vi "MAIN_load_previous_acquisition_data.vi"(3 "error in":errorcluster, 5 "Path to the saving folder":path=path "D:/MFM experiments") -> (0 "error out":errorcluster, 1 "Data cluster":T1, 2 "Menu names cluster":T2)   [LabVIEW 2015]
uses:
  GLOBAL/Global_MAIN.vi
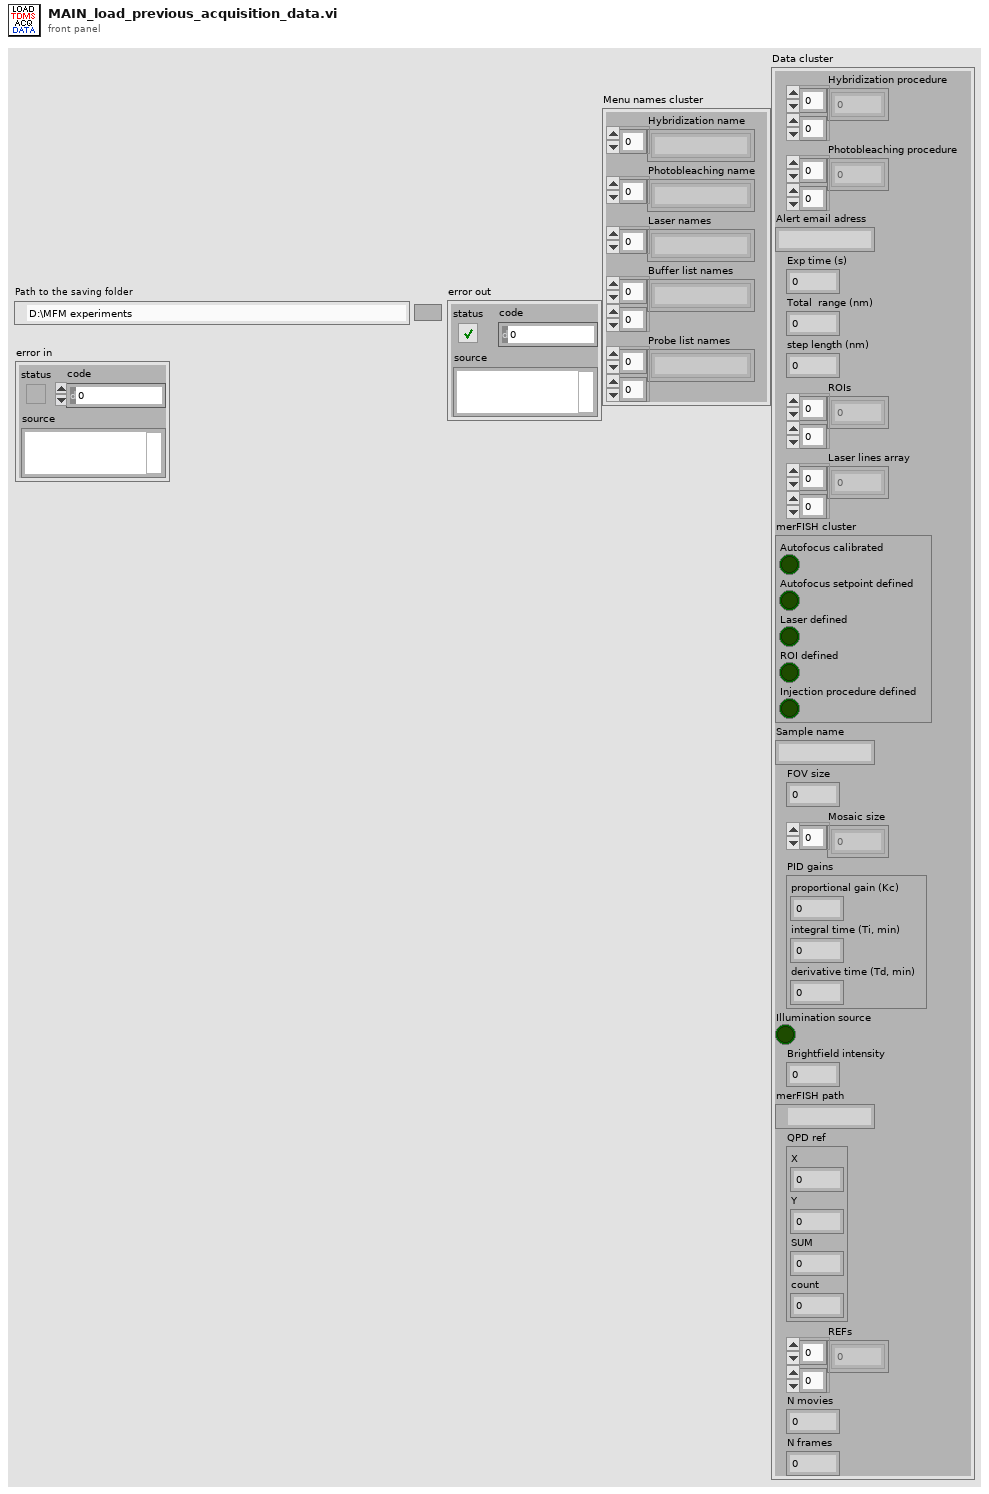
[diagram p1: front panel]
types:
  T1 = cluster{"Hybridization procedure":i32[][], "Photobleaching procedure":i32[][], "Alert email adress":string, "Exp time (s)":sgl, "Total  range (nm)":u32, "step length (nm)":u32, "ROIs":dbl[][], "Laser lines array":dbl[][], "merFISH cluster":cluster{"Autofocus calibrated":bool, "Autofocus setpoint defined":bool, "Laser defined":bool, "ROI defined":bool, "Injection procedure defined":bool}, "Sample name":string, "FOV size":dbl, "Mosaic size":u16[], "PID gains":cluster{"proportional gain (Kc)":dbl, "integral time (Ti, min)":dbl, "derivative time (Td, min)":dbl}, "Illumination source":bool, "Brightfield intensity":dbl, "merFISH path":path, "QPD ref":cluster{"X":sgl, "Y":sgl, "SUM":sgl, "count":u32}, "REFs":dbl[][], "N movies":i32, "N frames":i32}
  T2 = cluster{"Hybridization name":string[], "Photobleaching name":string[], "Laser names":string[], "Buffer list names":string[][], "Probe list names":string[][]}
  T3 = cluster{"X":sgl, "Y":sgl, "SUM":sgl, "count":u32}
  T4 = cluster{"proportional gain (Kc)":dbl, "integral time (Ti, min)":dbl, "derivative time (Td, min)":dbl}
  T5 = cluster{"Autofocus calibrated":bool, "Autofocus setpoint defined":bool, "Laser defined":bool, "ROI defined":bool, "Injection procedure defined":bool}
  T6 = enum16{"open", "open or create", "create or replace", "create", "open (read-only)"}
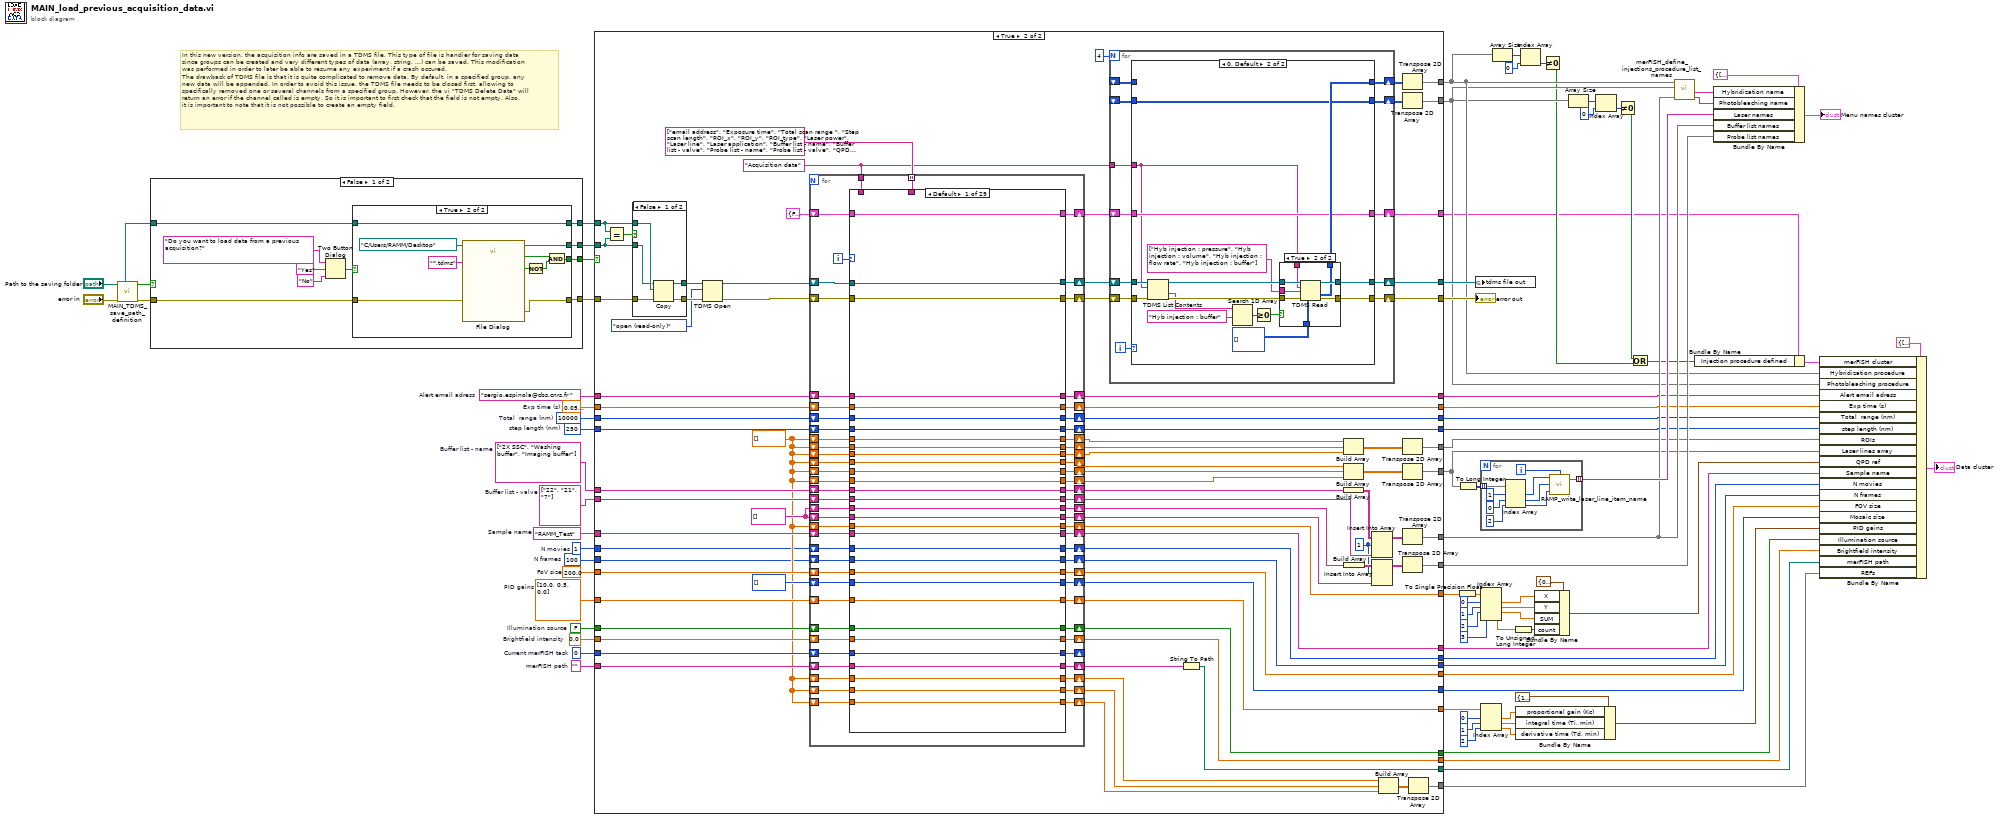
[diagram p0: block diagram]
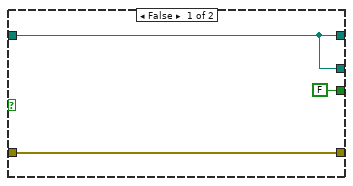
[diagram p2: hidden frame]
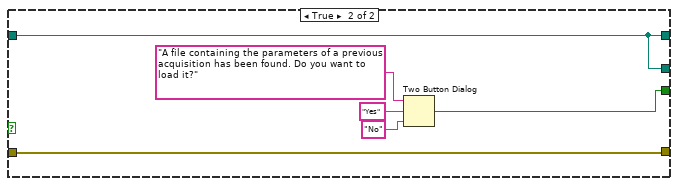
[diagram p3: hidden frame]
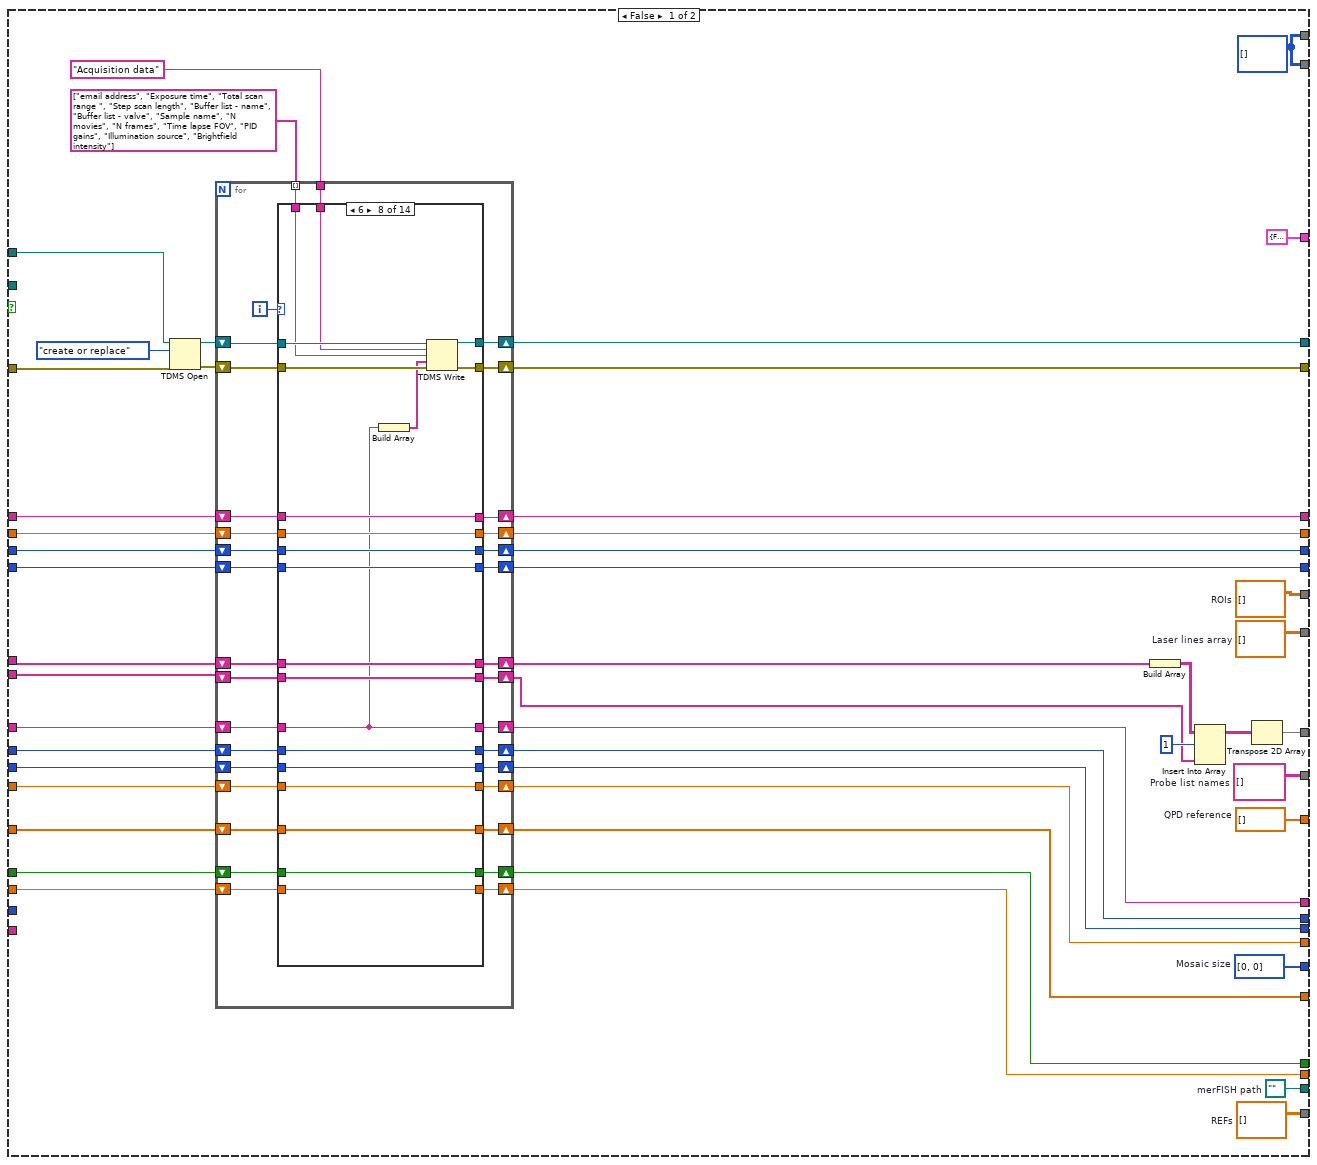
[diagram p4: hidden frame]
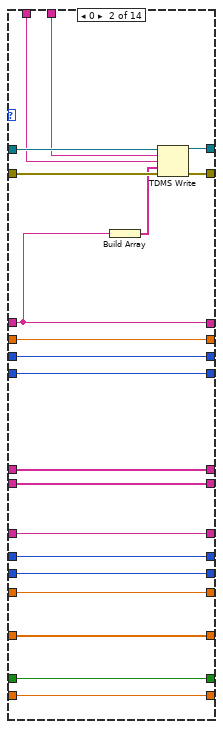
[diagram p6: hidden frame]
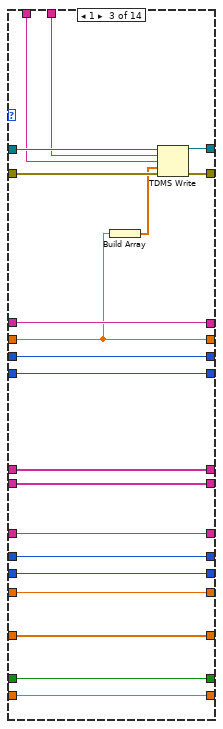
[diagram p7: hidden frame]
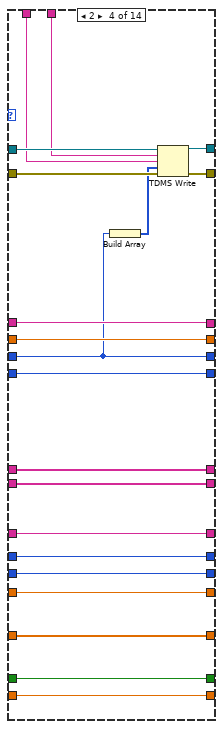
[diagram p8: hidden frame]
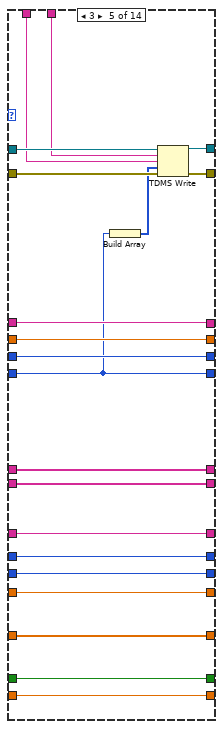
[diagram p9: hidden frame]
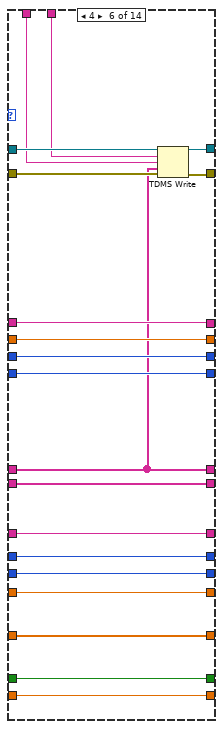
[diagram p10: hidden frame]
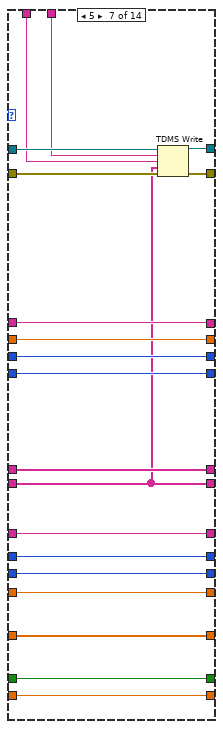
[diagram p11: hidden frame]
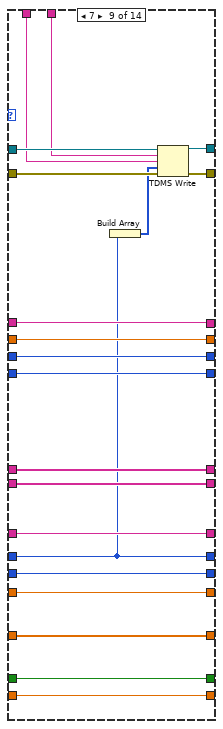
[diagram p12: hidden frame]
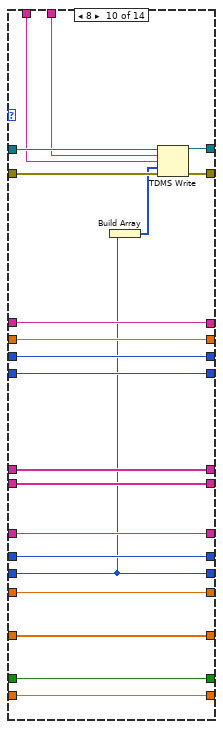
[diagram p13: hidden frame]
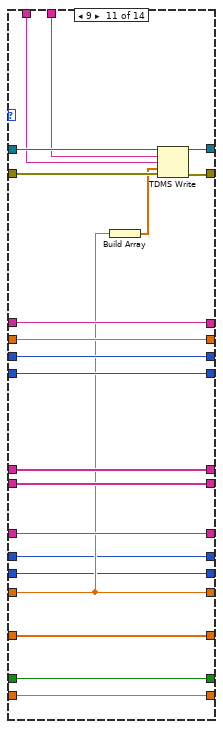
[diagram p14: hidden frame]
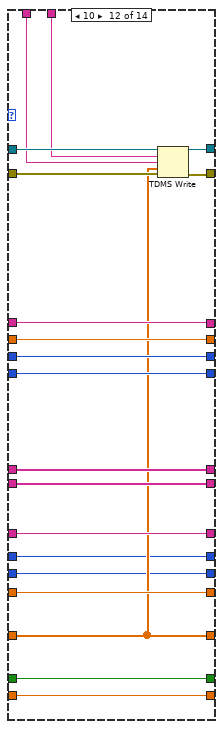
[diagram p15: hidden frame]
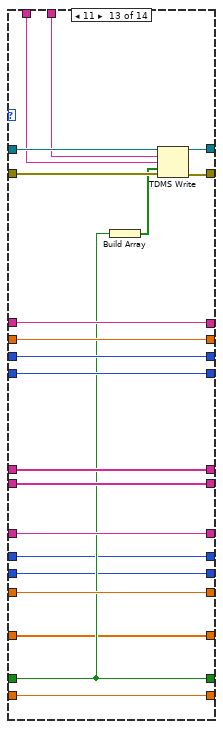
[diagram p16: hidden frame]
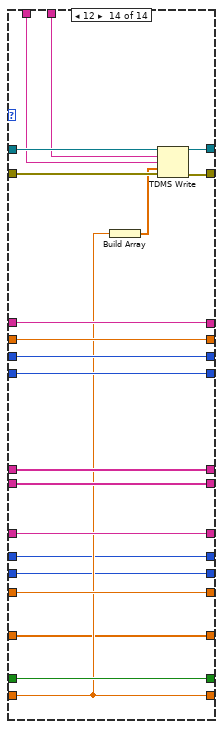
[diagram p17: hidden frame]
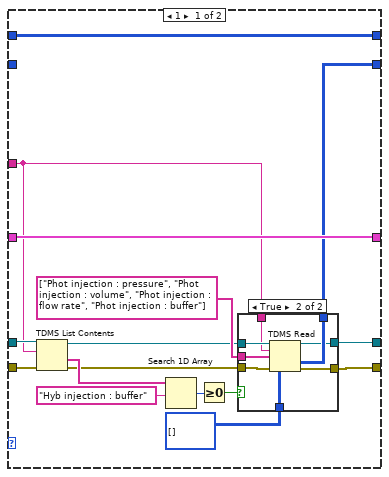
[diagram p18: hidden frame]
diagram:
  w12 = 100  # N frames
  w13 = 1  # N movies
  w19 = dbl[] [10.0, 0.5, 0.0]  # PID gains
  w21 = ""  # merFISH path
  w22 = u32 0  # Current merFISH task
  w23 = 0.0  # Brightfield intensity
  w24 = FALSE  # Illumination source
  w25 = 200.0  # FoV size
  w26 = "RAMM_Test"  # Sample name
  w27 = string[] ["22", "21", "7"]  # Buffer list - valve
  w28 = string[] ["2X SSC", "Washing buffer", "Imaging buffer"]  # Buffer list - name
  w32 = "sergio.espinola@cbs.cnrs.fr "  # Alert email adress
  w29 = u32 250  # step length (nm)
  w30 = u32 10000  # Total  range (nm)
  w31 = sgl 0.05  # Exp time (s)
  # "In this new version, the acquisition info are saved in a TDMS file. This type of file is handier for saving data\nsince groups can be created and very different types of data (array, string, ...) can be saved. This modification\nwas performed in order to later be able to resume any experiment if a crash occured.\nThe drawback of TDMS file is that it is quite complicated to remove data. By default, in a specified group, any\nnew data will be appended. In order to avoid this issue, the TDMS file needs to be closed first, allowing to \nspecifically removed one or several channels from a specified group. However, the vi \"TDMS Delete Data\" will\nreturn an error if the channel called is empty. So it is important to first check that the field is not empty. Also, \nit is important to note that it is not possible to create an empty field."
  n1 = call "MAIN_TDMS_save_path_definition.vi"("error in"="error in", "Path to the saving folder"="Path to the saving folder") -> ("error out"=w81:errorcluster, "file or folder exists?"=w82:bool, "path to tdms file"=w79:path)  [unwired: 4 in]
  n2 = case shown="False" w82 {
    tunnel: w81 -> [w93 w111]
    tunnel: [w92 w111] -> w80
    tunnel: [w91 w110] -> w78
    tunnel: [w90 w112] -> w77
    tunnel: w79 -> [w88 w110]
    tunnel: [w87 w110] -> w76
    frame False {
      n3 = Two Button Dialog(message="Do you want to load data from a previous acquisition?", 1:"No" ("Center Button Text (\"No\")"), 2:"Yes" ("Left Button Text (\"Yes\")")) -> (T button?=w89:bool)
      n4 = case shown="True" w89 {
        tunnel: w93 -> [w99 w104]
        tunnel: [w99 w103] -> w92
        tunnel: [w97 w101] -> w91
        tunnel: [FALSE w102] -> w90
        tunnel: w88 -> [w97 w101]
        tunnel: [w97 w100] -> w87
        frame False {
        }
        frame True {
          n5 = call "File Dialog"("start path"=path "C:/Users/RAMM/Desktop", "error in"=w104, "pattern (all files)"="*.tdms") -> ("selected path"=w100:path, "exists"=w106:bool, "cancelled"=w107:bool, "error out"=w103:errorcluster)  [unwired: 9 in]
          n6 = Not(x=w107) -> (.not. x?=w105:bool)
          n7 = And(x=w106, y=w105) -> (x .and. y?=w102:bool)
        }
      }
    }
    frame True {
      n8 = Two Button Dialog(message="A file containing the parameters of a previous acquisition has been found. Do you want to load it?", 1:"No" ("Center Button Text (\"No\")"), 2:"Yes" ("Left Button Text (\"Yes\")")) -> (T button?=w112:bool)
    }
  }
  n9 = case shown="True" w77 {
    tunnel: w80 -> [w162 w549]
    tunnel: [w131 w510] -> w85
    tunnel: [w130 w492] -> w86
    tunnel: w78 -> [w161 w548]
    tunnel: [w144 w540] -> w67
    tunnel: [w143 w539] -> w66
    tunnel: [w142 w537] -> w65
    tunnel: w76 -> [_ w547]
    tunnel: [w145 w541] -> w68
    tunnel: [w160 w529] -> w64
    tunnel: [w159 w524] -> w63
    tunnel: [w154 w522] -> w71
    tunnel: [w158 w520] -> w70
    tunnel: [w157 w535] -> w61
    tunnel: [w157 w534] -> w57
    tunnel: [T5 {"Autofocus calibrated"=FALSE, "Autofocus setpoint defined"=FALSE, "Laser defined"=FALSE, "ROI defined"=FALSE, "Injection procedure defined"=FALSE} ("merFISH init") w512] -> w51
    tunnel: [w155 w519] -> w49
    tunnel: [w138 w518] -> w41
    tunnel: [w136 w517] -> w3
    tunnel: [w153 w515] -> w4
    tunnel: [w126 w514] -> w34
    tunnel: w32 -> [w149 w507]
    tunnel: w31 -> [w148 w506]
    tunnel: w30 -> [w147 w505]
    tunnel: w29 -> [w146 w504]
    tunnel: w28 -> [w141 w503]
    tunnel: w27 -> [w140 w502]
    tunnel: w26 -> [w139 w501]
    tunnel: w25 -> [w137 w500]
    tunnel: w24 -> [w135 w488]
    tunnel: [w134 w487] -> w6
    tunnel: w23 -> [w133 w486]
    tunnel: [w132 w485] -> w7
    tunnel: w22 -> [_ w481]
    tunnel: w21 -> [_ w484]
    tunnel: [w129 w482] -> w8
    tunnel: w19 -> [w127 w480]
    tunnel: [w120 w473] -> w9
    tunnel: w13 -> [w119 w472]
    tunnel: w12 -> [w118 w471]
    tunnel: [w117 w469] -> w2
    tunnel: [w116 w470] -> w1
    frame False {
      w120 = dbl[][] []  # REFs
      w129 = path ""  # merFISH path
      w153 = u16[] [0, 0]  # Mosaic size
      w155 = dbl[] []  # QPD reference
      w157 = i32[][] []
      w158 = string[][] []  # Probe list names
      w159 = dbl[][] []  # Laser lines array
      w160 = dbl[][] []  # ROIs
      n10 = TDMS Open(8:w162, 10:T6."create or replace" ("operation (0:open)"), 11:w161) -> (0:w151:errorcluster, 3:w152:refnum<k34>)  [unwired: 4 in]
      n11 = for {
        shift-right: [w192] -> w130
        shift-left: w151 -> [w194]
        shift-right: [w191] -> w131
        shift-left: w152 -> [w193]
        shift-right: [w195] -> w145
        shift-left: w149 -> [w189]
        shift-right: [w190] -> w144
        shift-left: w148 -> [w188]
        shift-right: [w187] -> w143
        shift-left: w147 -> [w186]
        shift-right: [w184] -> w142
        shift-left: w146 -> [w185]
        shift-right: [w183] -> w124
        shift-left: w141 -> [w182]
        shift-right: [w180] -> w123
        shift-left: w140 -> [w181]
        tunnel: "Acquisition data" ("group name in") -> [w179]
        shift-right: [w177] -> w138
        shift-left: w139 -> [w178]
        shift-right: [w175] -> w136
        shift-left: w137 -> [w176]
        tunnel: string[] ["email address", "Exposure time", "Total scan range ", "Step scan length", "Buffer list - name", "Buffer list - valve", "Sample name", "N movies", "N frames", "Time lapse FOV", "PID gains", "Illumination source", "Brightfield intensity"] ("Buffer list - valve") -> [w174] mode=indexing
        shift-right: [w172] -> w134
        shift-left: w135 -> [w173]
        shift-right: [w170] -> w132
        shift-left: w133 -> [w171]
        shift-right: [w168] -> w126
        shift-left: w127 -> [w169]
        shift-right: [w166] -> w116
        shift-left: w119 -> [w167]
        shift-right: [w164] -> w117
        shift-left: w118 -> [w165]
        i -> [w196]
        n12 = case shown="6" w196 {
          tunnel: [w209 w217 w238 w259 w280 w301 w321 w339 w359 w379 w400 w420 w439 w459] -> w195
          tunnel: w174 -> [_ w221 w242 w263 w284 w304 w324 w343 w363 w383 w404 w423 w443 w463]
          tunnel: w194 -> [w210 w223 w244 w265 w286 w306 w326 w345 w365 w385 w406 w425 w445 w465]
          tunnel: w193 -> [w211 w224 w245 w266 w287 w307 w327 w346 w366 w386 w407 w426 w446 w466]
          tunnel: [w210 w219 w240 w261 w282 w303 w323 w341 w361 w381 w402 w422 w441 w461] -> w192
          tunnel: [w211 w218 w239 w260 w281 w302 w322 w340 w360 w380 w401 w421 w440 w460] -> w191
          tunnel: [w208 w231 w237 w258 w279 w300 w320 w338 w358 w378 w399 w419 w438 w458] -> w190
          tunnel: w189 -> [w209 w217 w238 w259 w280 w301 w321 w339 w359 w379 w400 w420 w439 w459]
          tunnel: w188 -> [w208 w231 w237 w258 w279 w300 w320 w338 w358 w378 w399 w419 w438 w458]
          tunnel: w186 -> [w207 w230 w251 w257 w278 w299 w319 w337 w357 w377 w398 w418 w437 w457]
          tunnel: [w207 w230 w251 w257 w278 w299 w319 w337 w357 w377 w398 w418 w437 w457] -> w187
          tunnel: w185 -> [w206 w229 w250 w271 w277 w298 w318 w336 w356 w376 w397 w417 w436 w456]
          tunnel: [w206 w229 w250 w271 w277 w298 w318 w336 w356 w376 w397 w417 w436 w456] -> w184
          tunnel: w182 -> [w205 w228 w249 w270 w291 w297 w317 w349 w369 w389 w409 w428 w448 w468]
          tunnel: [w205 w228 w249 w270 w291 w297 w317 w349 w369 w389 w409 w428 w448 w468] -> w183
          tunnel: w181 -> [w204 w227 w248 w269 w290 w310 w316 w348 w368 w388 w408 w427 w447 w467]
          tunnel: [w204 w227 w248 w269 w290 w310 w316 w348 w368 w388 w408 w427 w447 w467] -> w180
          tunnel: w179 -> [_ w222 w243 w264 w285 w305 w325 w344 w364 w384 w405 w424 w444 w464]
          tunnel: w178 -> [w203 w226 w247 w268 w289 w309 w329 w335 w355 w375 w396 w416 w435 w455]
          tunnel: [w203 w226 w247 w268 w289 w309 w329 w335 w355 w375 w396 w416 w435 w455] -> w177
          tunnel: w176 -> [w202 w225 w246 w267 w288 w308 w328 w347 w367 w387 w395 w415 w434 w454]
          tunnel: [w202 w225 w246 w267 w288 w308 w328 w347 w367 w387 w395 w415 w434 w454] -> w175
          tunnel: w173 -> [w201 w216 w236 w256 w276 w296 w315 w334 w354 w374 w394 w414 w433 w453]
          tunnel: [w201 w216 w236 w256 w276 w296 w315 w334 w354 w374 w394 w414 w433 w453] -> w172
          tunnel: w171 -> [w200 w215 w235 w255 w275 w295 w314 w333 w353 w373 w393 w413 w432 w452]
          tunnel: [w200 w215 w235 w255 w275 w295 w314 w333 w353 w373 w393 w413 w432 w452] -> w170
          tunnel: w169 -> [w199 w214 w234 w254 w274 w294 w313 w332 w352 w372 w392 w412 w431 w451]
          tunnel: [w199 w214 w234 w254 w274 w294 w313 w332 w352 w372 w392 w412 w431 w451] -> w168
          tunnel: w167 -> [w198 w213 w233 w253 w273 w293 w312 w331 w350 w371 w391 w411 w430 w450]
          tunnel: [w198 w213 w233 w253 w273 w293 w312 w331 w350 w371 w391 w411 w430 w450] -> w166
          tunnel: w165 -> [w197 w212 w232 w252 w272 w292 w311 w330 w351 w370 w390 w410 w429 w449]
          tunnel: [w197 w212 w232 w252 w272 w292 w311 w330 w351 w370 w390 w410 w429 w449] -> w164
          frame Default {
          }
          frame 0 {
            n13 = Build Array(w217) -> (w220:string[])
            n14 = TDMS Write(0:w224, 5:w222, 7:w221, 9:w220, 11:w223) -> (4:w218:refnum<k34>, 15:w219:errorcluster)  [unwired: 1 in, 2 out]
          }
          frame 1 {
            n15 = Build Array(w237) -> (w241:sgl[])
            n16 = TDMS Write(0:w245, 5:w243, 7:w242, 9:w241, 11:w244) -> (4:w239:refnum<k34>, 15:w240:errorcluster)  [unwired: 1 in, 2 out]
          }
          frame 2 {
            n17 = Build Array(w257) -> (w262:u32[])
            n18 = TDMS Write(0:w266, 5:w264, 7:w263, 9:w262, 11:w265) -> (4:w260:refnum<k34>, 15:w261:errorcluster)  [unwired: 1 in, 2 out]
          }
          frame 3 {
            n19 = Build Array(w277) -> (w283:u32[])
            n20 = TDMS Write(0:w287, 5:w285, 7:w284, 9:w283, 11:w286) -> (4:w281:refnum<k34>, 15:w282:errorcluster)  [unwired: 1 in, 2 out]
          }
          frame 4 {
            n21 = TDMS Write(0:w307, 5:w305, 7:w304, 9:w297, 11:w306) -> (4:w302:refnum<k34>, 15:w303:errorcluster)  [unwired: 1 in, 2 out]
          }
          frame 5 {
            n22 = TDMS Write(0:w327, 5:w325, 7:w324, 9:w316, 11:w326) -> (4:w322:refnum<k34>, 15:w323:errorcluster)  [unwired: 1 in, 2 out]
          }
          frame 6 {
            n23 = Build Array(w335) -> (w342:string[])
            n24 = TDMS Write(0:w346, 5:w344, 7:w343, 9:w342, 11:w345) -> (4:w340:refnum<k34>, 15:w341:errorcluster)  [unwired: 1 in, 2 out]
          }
          frame 7 {
            n25 = Build Array(w350) -> (w362:i32[])
            n26 = TDMS Write(0:w366, 5:w364, 7:w363, 9:w362, 11:w365) -> (4:w360:refnum<k34>, 15:w361:errorcluster)  [unwired: 1 in, 2 out]
          }
          frame 8 {
            n27 = Build Array(w370) -> (w382:i32[])
            n28 = TDMS Write(0:w386, 5:w384, 7:w383, 9:w382, 11:w385) -> (4:w380:refnum<k34>, 15:w381:errorcluster)  [unwired: 1 in, 2 out]
          }
          frame 9 {
            n29 = Build Array(w395) -> (w403:dbl[])
            n30 = TDMS Write(0:w407, 5:w405, 7:w404, 9:w403, 11:w406) -> (4:w401:refnum<k34>, 15:w402:errorcluster)  [unwired: 1 in, 2 out]
          }
          frame 10 {
            n31 = TDMS Write(0:w426, 5:w424, 7:w423, 9:w412, 11:w425) -> (4:w421:refnum<k34>, 15:w422:errorcluster)  [unwired: 1 in, 2 out]
          }
          frame 11 {
            n32 = Build Array(w433) -> (w442:bool[])
            n33 = TDMS Write(0:w446, 5:w444, 7:w443, 9:w442, 11:w445) -> (4:w440:refnum<k34>, 15:w441:errorcluster)  [unwired: 1 in, 2 out]
          }
          frame 12 {
            n34 = Build Array(w452) -> (w462:dbl[])
            n35 = TDMS Write(0:w466, 5:w464, 7:w463, 9:w462, 11:w465) -> (4:w460:refnum<k34>, 15:w461:errorcluster)  [unwired: 1 in, 2 out]
          }
        }
      }
      n36 = Build Array(w124) -> (w122:string[][])
      n37 = Insert Into Array(array=w122, index (row)=1, new element=w123) -> (w121:string[][])  [unwired: 1 in]
      n38 = Transpose 2D Array(2D array=w121) -> (transposed array=w154:string[][])
    }
    frame True {
      w493 = 1 ("index (row)")
      w536 = string[] [] ("ItemNames")
      w478 = dbl[] []
      w491 = "Acquisition data" ("group name in")
      n39 = Equal?(x=w548, y=w547) -> (x = y?=w550:bool)
      n40 = case shown="False" w550 {
        tunnel: w549 -> [w2218 w2219]
        tunnel: w548 -> [w2217 w2220]
        tunnel: w547 -> [w2216 _]
        tunnel: [w2215 w2219] -> w546
        tunnel: [w2214 w2220] -> w545
        frame False {
          n41 = Copy(8:w2218, 10:w2217, 11:w2216) -> (0:w2215:errorcluster, 3:w2214:path)  [unwired: 2 in, 1 out]
        }
        frame True {
        }
      }
      n42 = TDMS Open(8:w546, 10:T6."open (read-only)" ("operation (0:open)"), 11:w545) -> (0:w542:errorcluster, 3:w538:refnum<k34>)  [unwired: 4 in]
      n43 = for {
        tunnel: string[] ["email address", "Exposure time", "Total scan range ", "Step scan length", "ROI_x", "ROI_y", "ROI_type", "Laser power", "Laser line", "Laser application", "Buffer list - name", "Buffer list - valve", "Probe list - name", "Probe list - valve", "QPD reference", "Sample name", "N movies", "N frames", "Time lapse FOV", "Mosaic size", "PID gains", "Illumination source", "Brightfield intensity", "Current merFISH task number", "merFISH path", "Current TL task number", "REF_x", "REF_y", "REF_embryo"] ("channel name(s) in (Untitled)") -> [w679] mode=indexing
        shift-right: [w676] -> w509
        shift-left: w542 -> [w678]
        shift-right: [w675] -> w508
        shift-left: w538 -> [w677]
        shift-right: [w680] -> w541
        shift-left: w507 -> [w673]
        shift-right: [w674] -> w540
        shift-left: w506 -> [w672]
        shift-right: [w671] -> w539
        shift-left: w505 -> [w670]
        shift-right: [w668] -> w537
        shift-left: w504 -> [w669]
        shift-right: [w666] -> w532
        shift-left: w478 -> [w667]
        shift-right: [w664] -> w531
        shift-left: w478 -> [w665]
        shift-right: [w658] -> w528
        shift-left: w478 -> [w659]
        shift-right: [w662] -> w527
        shift-left: w478 -> [w663]
        shift-right: [w660] -> w526
        shift-left: w478 -> [w661]
        shift-right: [w657] -> w523
        shift-left: w503 -> [w656]
        shift-right: [w654] -> w498
        shift-left: w502 -> [w655]
        shift-right: [w651] -> w521
        shift-left: w536 -> [w653]
        shift-right: [w652] -> w494
        shift-left: w536 -> [w650]
        tunnel: w491 -> [w649]
        shift-right: [w647] -> w513
        shift-left: T5 {"Autofocus calibrated"=FALSE, "Autofocus setpoint defined"=FALSE, "Laser defined"=FALSE, "ROI defined"=FALSE, "Injection procedure defined"=FALSE} ("merFISH init") -> [w648]
        shift-right: [w645] -> w519
        shift-left: w478 -> [w646]
        shift-right: [w643] -> w518
        shift-left: w501 -> [w644]
        shift-right: [w641] -> w517
        shift-left: w500 -> [w642]
        shift-right: [w639] -> w515
        shift-left: u16[] [] -> [w640]
        shift-right: [w637] -> w514
        shift-left: w480 -> [w638]
        shift-right: [w635] -> w487
        shift-left: w488 -> [w636]
        shift-right: [w633] -> w485
        shift-left: w486 -> [w634]
        shift-right: [w631] -> w483
        shift-left: w484 -> [w632]
        shift-right: [w629] -> _
        shift-left: w481 -> [w630]
        shift-right: [w627] -> w479
        shift-left: w478 -> [w628]
        shift-right: [w625] -> w476
        shift-left: w478 -> [w626]
        shift-right: [w623] -> w475
        shift-left: w478 -> [w624]
        shift-right: [w621] -> w474
        shift-left: w478 -> [w622]
        shift-right: [w619] -> w470
        shift-left: w472 -> [w620]
        shift-right: [w617] -> w469
        shift-left: w471 -> [w618]
        i -> [w681]
        n44 = case shown="Default" w681 {
          tunnel: [w709 w752 w786 w844 w902 w962 w1014 w1066 w1121 w1174 w1227 w1279 w1332 w1385 w1447 w1500 w1531 w1586 w1641 w1696 w1756 w1808 w1855 w1910 w1965 w2020 w2073 w2125 w2177] -> w680
          tunnel: w679 -> [_ w736 w791 w849 w907 w967 w1019 w1071 w1126 w1179 w1232 w1284 w1337 w1390 w1427 w1482 w1539 w1594 w1649 w1704 w1761 w1813 w1863 w1918 w1973 w2028 w2080 w2132 w2184]
          tunnel: w678 -> [w710 w735 w790 w848 w906 w966 w1018 w1070 w1125 w1178 w1231 w1283 w1336 w1389 w1432 w1487 w1538 w1593 w1648 w1703 w1760 w1812 w1862 w1917 w1972 w2027 w2079 w2131 w2183]
          tunnel: w677 -> [w711 w734 w789 w847 w905 w965 w1017 w1069 w1124 w1177 w1230 w1282 w1335 w1388 w1433 w1488 w1537 w1592 w1647 w1702 w1759 w1811 w1861 w1916 w1971 w2026 w2078 w2130 w2182]
          tunnel: [w710 w732 w787 w845 w903 w963 w1015 w1067 w1122 w1175 w1228 w1280 w1333 w1386 w1449 w1502 w1535 w1590 w1645 w1700 w1757 w1809 w1859 w1914 w1969 w2024 w2076 w2128 w2180] -> w676
          tunnel: [w711 w733 w788 w846 w904 w964 w1016 w1068 w1123 w1176 w1229 w1281 w1334 w1387 w1448 w1501 w1536 w1591 w1646 w1701 w1758 w1810 w1860 w1915 w1970 w2025 w2077 w2129 w2181] -> w675
          tunnel: [w708 w756 w784 w843 w901 w961 w1013 w1065 w1120 w1173 w1226 w1278 w1331 w1384 w1446 w1499 w1557 w1612 w1667 w1722 w1755 w1807 w1881 w1936 w1991 w2046 w2098 w2150 w2202] -> w674
          tunnel: w673 -> [w709 w753 w786 w844 w902 w962 w1014 w1066 w1121 w1174 w1227 w1279 w1332 w1385 w1447 w1500 w1531 w1586 w1641 w1696 w1756 w1808 w1855 w1910 w1965 w2020 w2073 w2125 w2177]
          tunnel: w672 -> [w708 w756 w809 w843 w901 w961 w1013 w1065 w1120 w1173 w1226 w1278 w1331 w1384 w1446 w1499 w1557 w1612 w1667 w1722 w1755 w1807 w1881 w1936 w1991 w2046 w2098 w2150 w2202]
          tunnel: w670 -> [w707 w755 w808 w866 w900 w960 w1012 w1064 w1119 w1172 w1225 w1277 w1330 w1383 w1445 w1498 w1556 w1611 w1666 w1721 w1754 w1806 w1880 w1935 w1990 w2045 w2097 w2149 w2201]
          tunnel: [w707 w755 w808 w841 w900 w960 w1012 w1064 w1119 w1172 w1225 w1277 w1330 w1383 w1445 w1498 w1556 w1611 w1666 w1721 w1754 w1806 w1880 w1935 w1990 w2045 w2097 w2149 w2201] -> w671
          tunnel: w669 -> [w706 w754 w807 w865 w923 w959 w1011 w1063 w1118 w1171 w1224 w1276 w1329 w1382 w1444 w1497 w1555 w1610 w1665 w1720 w1753 w1805 w1879 w1934 w1989 w2044 w2096 w2148 w2200]
          tunnel: [w706 w754 w807 w865 w898 w959 w1011 w1063 w1118 w1171 w1224 w1276 w1329 w1382 w1444 w1497 w1555 w1610 w1665 w1720 w1753 w1805 w1879 w1934 w1989 w2044 w2096 w2148 w2200] -> w668
          tunnel: w667 -> [w705 w751 w806 w864 w922 w958 w1008 w1062 w1117 w1170 w1223 w1275 w1328 w1381 w1443 w1496 w1554 w1609 w1664 w1719 w1752 w1804 w1878 w1933 w1988 w2043 w2095 w2147 w2199]
          tunnel: [w705 w751 w806 w864 w922 w957 w1008 w1062 w1117 w1170 w1223 w1275 w1328 w1381 w1443 w1496 w1554 w1609 w1664 w1719 w1752 w1804 w1878 w1933 w1988 w2043 w2095 w2147 w2199] -> w666
          tunnel: w665 -> [w704 w750 w805 w863 w921 w980 w1010 w1049 w1114 w1169 w1222 w1274 w1327 w1380 w1442 w1495 w1553 w1608 w1663 w1718 w1747 w1799 w1877 w1932 w1987 w2042 w2094 w2146 w2198]
          tunnel: [w704 w750 w805 w863 w921 w980 w1009 w1049 w1114 w1169 w1222 w1274 w1327 w1380 w1442 w1495 w1553 w1608 w1663 w1718 w1747 w1799 w1877 w1932 w1987 w2042 w2094 w2146 w2198] -> w664
          tunnel: w663 -> [w702 w748 w803 w861 w919 w978 w1031 w1083 w1137 w1167 w1220 w1272 w1325 w1378 w1440 w1493 w1551 w1606 w1661 w1716 w1773 w1825 w1875 w1930 w1985 w2040 w2092 w2144 w2196]
          tunnel: [w702 w748 w803 w861 w919 w978 w1031 w1083 w1137 w1166 w1220 w1272 w1325 w1378 w1440 w1493 w1551 w1606 w1661 w1716 w1773 w1825 w1875 w1930 w1985 w2040 w2092 w2144 w2196] -> w662
          tunnel: w661 -> [w701 w747 w802 w860 w918 w977 w1030 w1082 w1136 w1165 w1218 w1269 w1324 w1377 w1439 w1492 w1550 w1605 w1660 w1715 w1772 w1824 w1874 w1929 w1984 w2039 w2091 w2143 w2195]
          tunnel: [w701 w747 w802 w860 w918 w977 w1030 w1082 w1136 w1165 w1217 w1269 w1324 w1377 w1439 w1492 w1550 w1605 w1660 w1715 w1772 w1824 w1874 w1929 w1984 w2039 w2091 w2143 w2195] -> w660
          tunnel: w659 -> [w703 w749 w804 w862 w920 w979 w1032 w1084 w1116 w1168 w1221 w1273 w1326 w1379 w1441 w1494 w1552 w1607 w1662 w1717 w1774 w1826 w1876 w1931 w1986 w2041 w2093 w2145 w2197]
          tunnel: [w703 w749 w804 w862 w920 w979 w1032 w1084 w1115 w1168 w1221 w1273 w1326 w1379 w1441 w1494 w1552 w1607 w1662 w1717 w1774 w1826 w1876 w1931 w1986 w2041 w2093 w2145 w2197] -> w658
          tunnel: w656 -> [w700 w746 w801 w859 w917 w976 w1029 w1081 w1135 w1189 w1219 w1271 w1321 w1376 w1438 w1491 w1549 w1604 w1659 w1714 w1771 w1823 w1873 w1928 w1983 w2038 w2090 w2142 w2194]
          tunnel: [w700 w746 w801 w859 w917 w976 w1029 w1081 w1135 w1189 w1219 w1270 w1321 w1376 w1438 w1491 w1549 w1604 w1659 w1714 w1771 w1823 w1873 w1928 w1983 w2038 w2090 w2142 w2194] -> w657
          tunnel: w655 -> [w699 w745 w800 w858 w916 w975 w1028 w1080 w1134 w1188 w1241 w1293 w1323 w1373 w1437 w1490 w1548 w1603 w1658 w1713 w1770 w1822 w1872 w1927 w1982 w2037 w2089 w2141 w2193]
          tunnel: [w699 w745 w800 w858 w916 w975 w1028 w1080 w1134 w1188 w1241 w1293 w1322 w1373 w1437 w1490 w1548 w1603 w1658 w1713 w1770 w1822 w1872 w1927 w1982 w2037 w2089 w2141 w2193] -> w654
          tunnel: w653 -> [w698 w744 w799 w857 w915 w974 w1027 w1079 w1133 w1187 w1240 w1292 w1345 w1375 w1436 w1489 w1547 w1602 w1657 w1712 w1769 w1821 w1871 w1926 w1981 w2036 w2088 w2140 w2192]
          tunnel: w650 -> [w697 w743 w798 w856 w914 w973 w1026 w1078 w1132 w1186 w1239 w1291 w1344 w1397 w1435 w1480 w1546 w1601 w1656 w1711 w1768 w1820 w1870 w1925 w1980 w2035 w2087 w2139 w2191]
          tunnel: [w697 w743 w798 w856 w914 w973 w1026 w1078 w1132 w1186 w1239 w1291 w1344 w1397 w1434 w1480 w1546 w1601 w1656 w1711 w1768 w1820 w1870 w1925 w1980 w2035 w2087 w2139 w2191] -> w652
          tunnel: [w698 w744 w799 w857 w915 w974 w1027 w1079 w1133 w1187 w1240 w1292 w1345 w1374 w1436 w1489 w1547 w1602 w1657 w1712 w1769 w1821 w1871 w1926 w1981 w2036 w2088 w2140 w2192] -> w651
          tunnel: w649 -> [_ w737 w792 w850 w908 w968 w1020 w1072 w1127 w1180 w1233 w1285 w1338 w1391 w1431 w1486 w1540 w1595 w1650 w1705 w1762 w1814 w1864 w1919 w1974 w2029 w2081 w2133 w2185]
          tunnel: w648 -> [w712 w728 w783 w840 w897 w956 w1007 w1061 w1113 w1164 w1216 w1268 w1320 w1372 w1424 w1476 w1533 w1588 w1643 w1698 w1751 w1803 w1857 w1912 w1967 w2022 w2075 w2127 w2179]
          tunnel: [w712 w728 w783 w840 w897 w954 w1007 w1061 w1111 w1164 w1216 w1268 w1320 w1372 w1424 w1475 w1533 w1588 w1643 w1698 w1751 w1803 w1857 w1912 w1967 w2022 w2075 w2127 w2179] -> w647
          tunnel: w646 -> [w696 w727 w782 w839 w896 w953 w1006 w1060 w1110 w1163 w1215 w1267 w1319 w1371 w1423 w1479 w1532 w1587 w1642 w1697 w1750 w1802 w1856 w1911 w1966 w2021 w2074 w2126 w2178]
          tunnel: [w696 w727 w782 w839 w896 w953 w1006 w1060 w1110 w1163 w1215 w1267 w1319 w1371 w1423 w1478 w1532 w1587 w1642 w1697 w1750 w1802 w1856 w1911 w1966 w2021 w2074 w2126 w2178] -> w645
          tunnel: w644 -> [w695 w726 w781 w838 w895 w952 w1005 w1059 w1109 w1162 w1214 w1266 w1318 w1370 w1422 w1474 w1530 w1571 w1627 w1694 w1749 w1801 w1853 w1908 w1963 w2018 w2072 w2124 w2176]
          tunnel: [w695 w726 w781 w838 w895 w952 w1005 w1059 w1109 w1162 w1214 w1266 w1318 w1370 w1422 w1474 w1527 w1571 w1627 w1694 w1749 w1801 w1853 w1908 w1963 w2018 w2072 w2124 w2176] -> w643
          tunnel: w642 -> [w694 w725 w780 w837 w894 w951 w1004 w1058 w1108 w1161 w1213 w1265 w1317 w1369 w1421 w1473 w1526 w1583 w1638 w1692 w1748 w1800 w1848 w1904 w1960 w2015 w2069 w2121 w2173]
          tunnel: [w694 w725 w780 w837 w894 w951 w1004 w1058 w1108 w1161 w1213 w1265 w1317 w1369 w1421 w1473 w1526 w1583 w1638 w1691 w1748 w1800 w1848 w1904 w1960 w2015 w2069 w2121 w2173] -> w641
          tunnel: w640 -> [w693 w724 w779 w836 w893 w950 w1003 w1057 w1107 w1160 w1212 w1264 w1316 w1368 w1420 w1472 w1525 w1582 w1637 w1690 w1746 w1796 w1851 w1906 w1962 w2017 w2071 w2123 w2175]
          tunnel: [w693 w724 w779 w836 w893 w950 w1003 w1057 w1107 w1160 w1212 w1264 w1316 w1368 w1420 w1472 w1525 w1582 w1637 w1690 w1745 w1796 w1851 w1906 w1962 w2017 w2071 w2123 w2175] -> w639
          tunnel: w638 -> [w692 w723 w778 w835 w892 w949 w1002 w1056 w1106 w1159 w1211 w1263 w1315 w1367 w1419 w1471 w1524 w1581 w1636 w1689 w1744 w1798 w1850 w1905 w1961 w2016 w2070 w2122 w2174]
          tunnel: [w692 w723 w778 w835 w892 w949 w1002 w1056 w1106 w1159 w1211 w1263 w1315 w1367 w1419 w1471 w1524 w1581 w1636 w1689 w1744 w1797 w1850 w1905 w1961 w2016 w2070 w2122 w2174] -> w637
          tunnel: w636 -> [w691 w722 w777 w834 w891 w948 w1001 w1055 w1105 w1158 w1210 w1262 w1314 w1366 w1418 w1470 w1523 w1580 w1635 w1688 w1743 w1795 w1849 w1901 w1959 w2014 w2068 w2120 w2172]
          tunnel: [w691 w722 w777 w834 w891 w948 w1001 w1055 w1105 w1158 w1210 w1262 w1314 w1366 w1418 w1470 w1523 w1580 w1635 w1688 w1743 w1795 w1847 w1901 w1959 w2014 w2068 w2120 w2172] -> w635
          tunnel: w634 -> [w690 w721 w776 w833 w890 w947 w1000 w1054 w1104 w1157 w1209 w1261 w1313 w1365 w1417 w1469 w1522 w1579 w1634 w1687 w1742 w1794 w1846 w1903 w1958 w2012 w2067 w2119 w2171]
          tunnel: [w690 w721 w776 w833 w890 w947 w1000 w1054 w1104 w1157 w1209 w1261 w1313 w1365 w1417 w1469 w1522 w1579 w1634 w1687 w1742 w1794 w1846 w1902 w1958 w2012 w2067 w2119 w2171] -> w633
          tunnel: w632 -> [w689 w720 w775 w832 w889 w946 w999 w1053 w1103 w1156 w1208 w1260 w1312 w1364 w1416 w1468 w1521 w1578 w1633 w1686 w1741 w1793 w1845 w1900 w1954 w2013 w2063 w2116 w2168]
          tunnel: [w689 w720 w775 w832 w889 w946 w999 w1053 w1103 w1156 w1208 w1260 w1312 w1364 w1416 w1468 w1521 w1578 w1633 w1686 w1741 w1793 w1845 w1900 w1954 w2010 w2063 w2116 w2168] -> w631
          tunnel: w630 -> [w688 w719 w774 w831 w888 w945 w998 w1052 w1102 w1155 w1207 w1259 w1311 w1363 w1415 w1467 w1520 w1577 w1632 w1685 w1740 w1792 w1844 w1899 w1957 w2009 w2066 w2118 w2170]
          tunnel: [w688 w719 w774 w831 w888 w945 w998 w1052 w1102 w1155 w1207 w1259 w1311 w1363 w1415 w1467 w1520 w1577 w1632 w1685 w1740 w1792 w1844 w1899 w1956 w2009 w2066 w2118 w2170] -> w629
          tunnel: w628 -> [w687 w718 w773 w830 w887 w944 w997 w1051 w1101 w1154 w1206 w1258 w1310 w1362 w1414 w1466 w1519 w1576 w1631 w1684 w1739 w1791 w1843 w1898 w1953 w2008 w2065 w2117 w2169]
          tunnel: [w687 w718 w773 w830 w887 w944 w997 w1050 w1101 w1154 w1206 w1258 w1310 w1362 w1414 w1466 w1519 w1576 w1631 w1684 w1739 w1791 w1843 w1898 w1953 w2008 w2065 w2117 w2169] -> w627
          tunnel: w626 -> [w686 w717 w772 w829 w886 w943 w996 w1048 w1100 w1153 w1205 w1257 w1309 w1361 w1413 w1465 w1518 w1575 w1630 w1683 w1738 w1790 w1842 w1897 w1952 w2007 w2064 w2112 w2167]
          tunnel: [w686 w717 w772 w829 w886 w943 w996 w1048 w1100 w1153 w1205 w1257 w1309 w1361 w1413 w1465 w1518 w1575 w1630 w1683 w1738 w1790 w1842 w1897 w1952 w2007 w2060 w2112 w2167] -> w625
          tunnel: w624 -> [w685 w716 w771 w828 w885 w942 w995 w1047 w1099 w1152 w1204 w1256 w1308 w1360 w1412 w1464 w1517 w1574 w1629 w1682 w1737 w1789 w1841 w1896 w1951 w2006 w2062 w2114 w2165]
          tunnel: [w685 w716 w771 w828 w885 w942 w995 w1047 w1099 w1152 w1204 w1256 w1308 w1360 w1412 w1464 w1517 w1574 w1629 w1682 w1737 w1789 w1841 w1896 w1951 w2006 w2062 w2113 w2165] -> w623
          tunnel: w622 -> [w684 w715 w770 w827 w884 w941 w994 w1046 w1098 w1151 w1203 w1255 w1307 w1359 w1411 w1463 w1516 w1573 w1628 w1681 w1736 w1788 w1840 w1895 w1950 w2005 w2061 w2115 w2166]
          tunnel: [w684 w715 w770 w827 w884 w941 w994 w1046 w1098 w1151 w1203 w1255 w1307 w1359 w1411 w1463 w1516 w1573 w1628 w1681 w1736 w1788 w1840 w1895 w1950 w2005 w2061 w2115 w2164] -> w621
          tunnel: w620 -> [w683 w714 w769 w826 w883 w940 w993 w1045 w1097 w1150 w1202 w1254 w1306 w1358 w1410 w1462 w1515 w1572 w1624 w1680 w1735 w1787 w1839 w1894 w1949 w2004 w2059 w2111 w2163]
          tunnel: [w683 w714 w769 w826 w883 w940 w993 w1045 w1097 w1150 w1202 w1254 w1306 w1358 w1410 w1462 w1515 w1570 w1624 w1680 w1735 w1787 w1839 w1894 w1949 w2004 w2059 w2111 w2163] -> w619
          tunnel: [w682 w713 w768 w825 w882 w939 w992 w1044 w1096 w1149 w1201 w1253 w1305 w1357 w1409 w1461 w1514 w1569 w1625 w1679 w1734 w1786 w1838 w1893 w1948 w2003 w2058 w2110 w2162] -> w617
          tunnel: w618 -> [w682 w713 w768 w825 w882 w939 w992 w1044 w1096 w1149 w1201 w1253 w1305 w1357 w1409 w1461 w1514 w1569 w1626 w1679 w1734 w1786 w1838 w1893 w1948 w2003 w2058 w2110 w2162]
          frame Default {
          }
          frame 0 {
            n45 = TDMS List Contents(4:w735, 6:w737, 7:w734) -> (0:w741:errorcluster, 1:w740:string[], 3:w742:refnum<k34>)  [unwired: 1 out]
            n46 = Build Array(w753) -> (w730:string[])
            n47 = Search 1D Array(1D array=w740, element=w736) -> (index of element=w739:i32)  [unwired: 1 in]
            n48 = Greater Or Equal To 0?(x=w739) -> (x >= 0?=w738:bool)
            n49 = case shown="True" w738 {
              tunnel: [w758 w763] -> w732
              tunnel: [w759 w767] -> w733
              tunnel: w737 -> [_ w761]
              tunnel: w742 -> [w759 w766]
              tunnel: w741 -> [w758 w765]
              tunnel: w736 -> [_ w760]
              tunnel: w730 -> [w757 w764]
              tunnel: [w757 w762] -> w729
              frame False {
              }
              frame True {
                n50 = TDMS Read(0:w766, 5:w761, 7:w760, 11:w765, 12:w764) -> (4:w767:refnum<k34>, 10:w762:string[], 15:w763:errorcluster)  [unwired: 3 in, 3 out]
              }
            }
            n51 = Index Array(array=w729, index=0) -> (element=w752:string)
          }
          frame 1 {
            n52 = TDMS List Contents(4:w790, 6:w792, 7:w789) -> (0:w796:errorcluster, 1:w795:string[], 3:w797:refnum<k34>)  [unwired: 1 out]
            n53 = Build Array(w809) -> (w785:sgl[])
            n54 = Search 1D Array(1D array=w795, element=w791) -> (index of element=w794:i32)  [unwired: 1 in]
            n55 = Greater Or Equal To 0?(x=w794) -> (x >= 0?=w793:bool)
            n56 = case shown="True" w793 {
              tunnel: [w813 w820] -> w787
              tunnel: [w814 w824] -> w788
              tunnel: w792 -> [_ w818]
              tunnel: w797 -> [w814 w823]
              tunnel: w796 -> [w813 w822]
              tunnel: w791 -> [_ w819]
              tunnel: w785 -> [w811 w821]
              tunnel: [w812 w815] -> w784
              frame False {
                n57 = Index Array(array=w811, index=0) -> (element=w812:sgl)
              }
              frame True {
                n58 = TDMS Read(0:w823, 5:w818, 7:w819, 11:w822, 12:w821) -> (4:w824:refnum<k34>, 10:w817:sgl[], 15:w820:errorcluster)  [unwired: 3 in, 3 out]
                n59 = Index Array(array=w817, index=0) -> (element=w815:sgl)
              }
            }
          }
          frame 2 {
            n60 = TDMS List Contents(4:w848, 6:w850, 7:w847) -> (0:w854:errorcluster, 1:w853:string[], 3:w855:refnum<k34>)  [unwired: 1 out]
            n61 = Build Array(w866) -> (w842:u32[])
            n62 = Search 1D Array(1D array=w853, element=w849) -> (index of element=w852:i32)  [unwired: 1 in]
            n63 = Greater Or Equal To 0?(x=w852) -> (x >= 0?=w851:bool)
            n64 = case shown="True" w851 {
              tunnel: [w870 w877] -> w845
              tunnel: [w871 w881] -> w846
              tunnel: w850 -> [_ w875]
              tunnel: w855 -> [w871 w880]
              tunnel: w854 -> [w870 w879]
              tunnel: w849 -> [_ w876]
              tunnel: w842 -> [w868 w878]
              tunnel: [w869 w872] -> w841
              frame False {
                n65 = Index Array(array=w868, index=0) -> (element=w869:u32)
              }
              frame True {
                n66 = TDMS Read(0:w880, 5:w875, 7:w876, 11:w879, 12:w878) -> (4:w881:refnum<k34>, 10:w874:u32[], 15:w877:errorcluster)  [unwired: 3 in, 3 out]
                n67 = Index Array(array=w874, index=0) -> (element=w872:u32)
              }
            }
          }
          frame 3 {
            n68 = TDMS List Contents(4:w906, 6:w908, 7:w905) -> (0:w912:errorcluster, 1:w911:string[], 3:w913:refnum<k34>)  [unwired: 1 out]
            n69 = Build Array(w923) -> (w899:u32[])
            n70 = Search 1D Array(1D array=w911, element=w907) -> (index of element=w910:i32)  [unwired: 1 in]
            n71 = Greater Or Equal To 0?(x=w910) -> (x >= 0?=w909:bool)
            n72 = case shown="True" w909 {
              tunnel: [w927 w934] -> w903
              tunnel: [w928 w938] -> w904
              tunnel: w908 -> [_ w932]
              tunnel: w913 -> [w928 w937]
              tunnel: w912 -> [w927 w936]
              tunnel: w907 -> [_ w933]
              tunnel: w899 -> [w925 w935]
              tunnel: [w926 w929] -> w898
              frame False {
                n73 = Index Array(array=w925, index=0) -> (element=w926:u32)
              }
              frame True {
                n74 = TDMS Read(0:w937, 5:w932, 7:w933, 11:w936, 12:w935) -> (4:w938:refnum<k34>, 10:w931:u32[], 15:w934:errorcluster)  [unwired: 3 in, 3 out]
                n75 = Index Array(array=w931, index=0) -> (element=w929:u32)
              }
            }
          }
          frame 4 {
            n76 = TDMS List Contents(4:w966, 6:w968, 7:w965) -> (0:w971:errorcluster, 1:w970:string[], 3:w972:refnum<k34>)  [unwired: 1 out]
            n77 = Search 1D Array(1D array=w970, element=w967) -> (index of element=w969:i32)  [unwired: 1 in]
            n78 = Greater Or Equal To 0?(x=w969) -> (x >= 0?=w955:bool)
            n79 = Bundle By Name(cluster=w956, "ROI defined"=w955) -> (w954:T5)
            n80 = case shown="True" w955 {
              tunnel: [w982 w987] -> w963
              tunnel: [w983 w991] -> w964
              tunnel: w968 -> [_ w985]
              tunnel: w972 -> [w983 w990]
              tunnel: w971 -> [w982 w989]
              tunnel: w967 -> [_ w986]
              tunnel: w958 -> [w981 w988]
              tunnel: [w981 w984] -> w957
              frame False {
              }
              frame True {
                n81 = TDMS Read(0:w990, 5:w985, 7:w986, 11:w989, 12:w988) -> (4:w991:refnum<k34>, 10:w984:dbl[], 15:w987:errorcluster)  [unwired: 3 in, 3 out]
              }
            }
          }
          frame 5 {
            n82 = TDMS List Contents(4:w1018, 6:w1020, 7:w1017) -> (0:w1024:errorcluster, 1:w1023:string[], 3:w1025:refnum<k34>)  [unwired: 1 out]
            n83 = Search 1D Array(1D array=w1023, element=w1019) -> (index of element=w1022:i32)  [unwired: 1 in]
            n84 = Greater Or Equal To 0?(x=w1022) -> (x >= 0?=w1021:bool)
            n85 = case shown="True" w1021 {
              tunnel: [w1034 w1039] -> w1015
              tunnel: [w1035 w1043] -> w1016
              tunnel: w1020 -> [_ w1037]
              tunnel: w1025 -> [w1035 w1042]
              tunnel: w1024 -> [w1034 w1041]
              tunnel: w1019 -> [_ w1038]
              tunnel: w1010 -> [w1033 w1040]
              tunnel: [w1033 w1036] -> w1009
              frame False {
              }
              frame True {
                n86 = TDMS Read(0:w1042, 5:w1037, 7:w1038, 11:w1041, 12:w1040) -> (4:w1043:refnum<k34>, 10:w1036:dbl[], 15:w1039:errorcluster)  [unwired: 3 in, 3 out]
              }
            }
          }
          frame 6 {
            n87 = TDMS List Contents(4:w1070, 6:w1072, 7:w1069) -> (0:w1076:errorcluster, 1:w1075:string[], 3:w1077:refnum<k34>)  [unwired: 1 out]
            n88 = Search 1D Array(1D array=w1075, element=w1071) -> (index of element=w1074:i32)  [unwired: 1 in]
            n89 = Greater Or Equal To 0?(x=w1074) -> (x >= 0?=w1073:bool)
            n90 = case shown="True" w1073 {
              tunnel: [w1086 w1091] -> w1067
              tunnel: [w1087 w1095] -> w1068
              tunnel: w1072 -> [_ w1089]
              tunnel: w1077 -> [w1087 w1094]
              tunnel: w1076 -> [w1086 w1093]
              tunnel: w1071 -> [_ w1090]
              tunnel: w1051 -> [w1085 w1092]
              tunnel: [w1085 w1088] -> w1050
              frame False {
              }
              frame True {
                n91 = TDMS Read(0:w1094, 5:w1089, 7:w1090, 11:w1093, 12:w1092) -> (4:w1095:refnum<k34>, 10:w1088:dbl[], 15:w1091:errorcluster)  [unwired: 3 in, 3 out]
              }
            }
          }
          frame 7 {
            n92 = TDMS List Contents(4:w1125, 6:w1127, 7:w1124) -> (0:w1130:errorcluster, 1:w1129:string[], 3:w1131:refnum<k34>)  [unwired: 1 out]
            n93 = Search 1D Array(1D array=w1129, element=w1126) -> (index of element=w1128:i32)  [unwired: 1 in]
            n94 = Greater Or Equal To 0?(x=w1128) -> (x >= 0?=w1112:bool)
            n95 = case shown="True" w1112 {
              tunnel: [w1139 w1144] -> w1122
              tunnel: [w1140 w1148] -> w1123
              tunnel: w1127 -> [_ w1142]
              tunnel: w1131 -> [w1140 w1147]
              tunnel: w1130 -> [w1139 w1146]
              tunnel: w1126 -> [_ w1143]
              tunnel: w1116 -> [w1138 w1145]
              tunnel: [w1138 w1141] -> w1115
              frame False {
              }
              frame True {
                n96 = TDMS Read(0:w1147, 5:w1142, 7:w1143, 11:w1146, 12:w1145) -> (4:w1148:refnum<k34>, 10:w1141:dbl[], 15:w1144:errorcluster)  [unwired: 3 in, 3 out]
              }
            }
            n97 = Bundle By Name(cluster=w1113, "Laser defined"=w1112) -> (w1111:T5)
          }
          frame 8 {
            n98 = TDMS List Contents(4:w1178, 6:w1180, 7:w1177) -> (0:w1184:errorcluster, 1:w1183:string[], 3:w1185:refnum<k34>)  [unwired: 1 out]
            n99 = Search 1D Array(1D array=w1183, element=w1179) -> (index of element=w1182:i32)  [unwired: 1 in]
            n100 = Greater Or Equal To 0?(x=w1182) -> (x >= 0?=w1181:bool)
            n101 = case shown="True" w1181 {
              tunnel: [w1191 w1196] -> w1175
              tunnel: [w1192 w1200] -> w1176
              tunnel: w1180 -> [_ w1194]
              tunnel: w1185 -> [w1192 w1199]
              tunnel: w1184 -> [w1191 w1198]
              tunnel: w1179 -> [_ w1195]
              tunnel: w1167 -> [w1190 w1197]
              tunnel: [w1190 w1193] -> w1166
              frame False {
              }
              frame True {
                n102 = TDMS Read(0:w1199, 5:w1194, 7:w1195, 11:w1198, 12:w1197) -> (4:w1200:refnum<k34>, 10:w1193:dbl[], 15:w1196:errorcluster)  [unwired: 3 in, 3 out]
              }
            }
          }
          frame 9 {
            n103 = TDMS List Contents(4:w1231, 6:w1233, 7:w1230) -> (0:w1237:errorcluster, 1:w1236:string[], 3:w1238:refnum<k34>)  [unwired: 1 out]
            n104 = Search 1D Array(1D array=w1236, element=w1232) -> (index of element=w1235:i32)  [unwired: 1 in]
            n105 = Greater Or Equal To 0?(x=w1235) -> (x >= 0?=w1234:bool)
            n106 = case shown="True" w1234 {
              tunnel: [w1243 w1248] -> w1228
              tunnel: [w1244 w1252] -> w1229
              tunnel: w1233 -> [_ w1246]
              tunnel: w1238 -> [w1244 w1251]
              tunnel: w1237 -> [w1243 w1250]
              tunnel: w1232 -> [_ w1247]
              tunnel: w1218 -> [w1242 w1249]
              tunnel: [w1242 w1245] -> w1217
              frame False {
              }
              frame True {
                n107 = TDMS Read(0:w1251, 5:w1246, 7:w1247, 11:w1250, 12:w1249) -> (4:w1252:refnum<k34>, 10:w1245:dbl[], 15:w1248:errorcluster)  [unwired: 3 in, 3 out]
              }
            }
          }
          frame 10 {
            n108 = TDMS List Contents(4:w1283, 6:w1285, 7:w1282) -> (0:w1289:errorcluster, 1:w1288:string[], 3:w1290:refnum<k34>)  [unwired: 1 out]
            n109 = Search 1D Array(1D array=w1288, element=w1284) -> (index of element=w1287:i32)  [unwired: 1 in]
            n110 = Greater Or Equal To 0?(x=w1287) -> (x >= 0?=w1286:bool)
            n111 = case shown="True" w1286 {
              tunnel: [w1295 w1300] -> w1280
              tunnel: [w1296 w1304] -> w1281
              tunnel: w1285 -> [_ w1298]
              tunnel: w1290 -> [w1296 w1303]
              tunnel: w1289 -> [w1295 w1302]
              tunnel: w1284 -> [_ w1299]
              tunnel: w1271 -> [w1294 w1301]
              tunnel: [w1294 w1297] -> w1270
              frame False {
              }
              frame True {
                n112 = TDMS Read(0:w1303, 5:w1298, 7:w1299, 11:w1302, 12:w1301) -> (4:w1304:refnum<k34>, 10:w1297:string[], 15:w1300:errorcluster)  [unwired: 3 in, 3 out]
              }
            }
          }
          frame 11 {
            n113 = TDMS List Contents(4:w1336, 6:w1338, 7:w1335) -> (0:w1342:errorcluster, 1:w1341:string[], 3:w1343:refnum<k34>)  [unwired: 1 out]
            n114 = Search 1D Array(1D array=w1341, element=w1337) -> (index of element=w1340:i32)  [unwired: 1 in]
            n115 = Greater Or Equal To 0?(x=w1340) -> (x >= 0?=w1339:bool)
            n116 = case shown="True" w1339 {
              tunnel: [w1347 w1352] -> w1333
              tunnel: [w1348 w1356] -> w1334
              tunnel: w1338 -> [_ w1350]
              tunnel: w1343 -> [w1348 w1355]
              tunnel: w1342 -> [w1347 w1354]
              tunnel: w1337 -> [_ w1351]
              tunnel: w1323 -> [w1346 w1353]
              tunnel: [w1346 w1349] -> w1322
              frame False {
              }
              frame True {
                n117 = TDMS Read(0:w1355, 5:w1350, 7:w1351, 11:w1354, 12:w1353) -> (4:w1356:refnum<k34>, 10:w1349:string[], 15:w1352:errorcluster)  [unwired: 3 in, 3 out]
              }
            }
          }
          frame 12 {
            n118 = TDMS List Contents(4:w1389, 6:w1391, 7:w1388) -> (0:w1395:errorcluster, 1:w1394:string[], 3:w1396:refnum<k34>)  [unwired: 1 out]
            n119 = Search 1D Array(1D array=w1394, element=w1390) -> (index of element=w1393:i32)  [unwired: 1 in]
            n120 = Greater Or Equal To 0?(x=w1393) -> (x >= 0?=w1392:bool)
            n121 = case shown="False" w1392 {
              tunnel: [w1399 w1404] -> w1386
              tunnel: [w1400 w1408] -> w1387
              tunnel: w1391 -> [_ w1402]
              tunnel: w1396 -> [w1400 w1407]
              tunnel: w1395 -> [w1399 w1406]
              tunnel: w1390 -> [_ w1403]
              tunnel: w1375 -> [w1398 w1405]
              tunnel: [w1398 w1401] -> w1374
              frame False {
              }
              frame True {
                n122 = TDMS Read(0:w1407, 5:w1402, 7:w1403, 11:w1406, 12:w1405) -> (4:w1408:refnum<k34>, 10:w1401:string[], 15:w1404:errorcluster)  [unwired: 3 in, 3 out]
              }
            }
          }
          frame 13 {
            n123 = TDMS List Contents(4:w1432, 6:w1431, 7:w1433) -> (0:w1429:errorcluster, 1:w1428:string[], 3:w1430:refnum<k34>)  [unwired: 1 out]
            n124 = Search 1D Array(1D array=w1428, element=w1427) -> (index of element=w1426:i32)  [unwired: 1 in]
            n125 = Greater Or Equal To 0?(x=w1426) -> (x >= 0?=w1425:bool)
            n126 = case shown="False" w1425 {
              tunnel: [w1451 w1460] -> w1449
              tunnel: [w1452 w1459] -> w1448
              tunnel: w1435 -> [w1450 w1458]
              tunnel: [w1450 w1457] -> w1434
              tunnel: w1431 -> [_ w1456]
              tunnel: w1430 -> [w1452 w1455]
              tunnel: w1429 -> [w1451 w1454]
              tunnel: w1427 -> [_ w1453]
              frame False {
              }
              frame True {
                n127 = TDMS Read(0:w1455, 5:w1456, 7:w1453, 11:w1454, 12:w1458) -> (4:w1459:refnum<k34>, 10:w1457:string[], 15:w1460:errorcluster)  [unwired: 3 in, 3 out]
              }
            }
          }
          frame 14 {
            n128 = TDMS List Contents(4:w1487, 6:w1486, 7:w1488) -> (0:w1484:errorcluster, 1:w1483:string[], 3:w1485:refnum<k34>)  [unwired: 1 out]
            n129 = Search 1D Array(1D array=w1483, element=w1482) -> (index of element=w1481:i32)  [unwired: 1 in]
            n130 = Greater Or Equal To 0?(x=w1481) -> (x >= 0?=w1477:bool)
            n131 = Bundle By Name(cluster=w1476, "Autofocus setpoint defined"=w1477) -> (w1475:T5)
            n132 = case shown="True" w1477 {
              tunnel: [w1504 w1513] -> w1502
              tunnel: [w1505 w1512] -> w1501
              tunnel: w1479 -> [w1503 w1511]
              tunnel: [w1503 w1510] -> w1478
              tunnel: w1486 -> [_ w1509]
              tunnel: w1485 -> [w1505 w1508]
              tunnel: w1484 -> [w1504 w1507]
              tunnel: w1482 -> [_ w1506]
              frame False {
              }
              frame True {
                n133 = TDMS Read(0:w1508, 5:w1509, 7:w1506, 11:w1507, 12:w1511) -> (4:w1512:refnum<k34>, 10:w1510:dbl[], 15:w1513:errorcluster)  [unwired: 3 in, 3 out]
              }
            }
          }
          frame 15 {
            n134 = TDMS List Contents(4:w1538, 6:w1540, 7:w1537) -> (0:w1544:errorcluster, 1:w1543:string[], 3:w1545:refnum<k34>)  [unwired: 1 out]
            n135 = Build Array(w1530) -> (w1529:string[])
            n136 = Search 1D Array(1D array=w1543, element=w1539) -> (index of element=w1542:i32)  [unwired: 1 in]
            n137 = Greater Or Equal To 0?(x=w1542) -> (x >= 0?=w1541:bool)
            n138 = case shown="True" w1541 {
              tunnel: [w1559 w1564] -> w1535
              tunnel: [w1560 w1568] -> w1536
              tunnel: w1540 -> [_ w1562]
              tunnel: w1545 -> [w1560 w1567]
              tunnel: w1544 -> [w1559 w1566]
              tunnel: w1539 -> [_ w1561]
              tunnel: w1529 -> [w1558 w1565]
              tunnel: [w1558 w1563] -> w1528
              frame False {
              }
              frame True {
                n139 = TDMS Read(0:w1567, 5:w1562, 7:w1561, 11:w1566, 12:w1565) -> (4:w1568:refnum<k34>, 10:w1563:string[], 15:w1564:errorcluster)  [unwired: 3 in, 3 out]
              }
            }
            n140 = Index Array(array=w1528, index=0) -> (element=w1527:string)
          }
          frame 16 {
            n141 = TDMS List Contents(4:w1593, 6:w1595, 7:w1592) -> (0:w1599:errorcluster, 1:w1598:string[], 3:w1600:refnum<k34>)  [unwired: 1 out]
            n142 = Build Array(w1572) -> (w1585:i32[])
            n143 = Search 1D Array(1D array=w1598, element=w1594) -> (index of element=w1597:i32)  [unwired: 1 in]
            n144 = Greater Or Equal To 0?(x=w1597) -> (x >= 0?=w1596:bool)
            n145 = case shown="True" w1596 {
              tunnel: [w1614 w1619] -> w1590
              tunnel: [w1615 w1623] -> w1591
              tunnel: w1595 -> [_ w1617]
              tunnel: w1600 -> [w1615 w1622]
              tunnel: w1599 -> [w1614 w1621]
              tunnel: w1594 -> [_ w1616]
              tunnel: w1585 -> [w1613 w1620]
              tunnel: [w1613 w1618] -> w1584
              frame False {
              }
              frame True {
                n146 = TDMS Read(0:w1622, 5:w1617, 7:w1616, 11:w1621, 12:w1620) -> (4:w1623:refnum<k34>, 10:w1618:i32[], 15:w1619:errorcluster)  [unwired: 3 in, 3 out]
              }
            }
            n147 = Index Array(array=w1584, index=0) -> (element=w1570:i32)
          }
          frame 17 {
            n148 = TDMS List Contents(4:w1648, 6:w1650, 7:w1647) -> (0:w1654:errorcluster, 1:w1653:string[], 3:w1655:refnum<k34>)  [unwired: 1 out]
            n149 = Build Array(w1626) -> (w1640:i32[])
            n150 = Search 1D Array(1D array=w1653, element=w1649) -> (index of element=w1652:i32)  [unwired: 1 in]
            n151 = Greater Or Equal To 0?(x=w1652) -> (x >= 0?=w1651:bool)
            n152 = case shown="True" w1651 {
              tunnel: [w1669 w1674] -> w1645
              tunnel: [w1670 w1678] -> w1646
              tunnel: w1650 -> [_ w1672]
              tunnel: w1655 -> [w1670 w1677]
              tunnel: w1654 -> [w1669 w1676]
              tunnel: w1649 -> [_ w1671]
              tunnel: w1640 -> [w1668 w1675]
              tunnel: [w1668 w1673] -> w1639
              frame False {
              }
              frame True {
                n153 = TDMS Read(0:w1677, 5:w1672, 7:w1671, 11:w1676, 12:w1675) -> (4:w1678:refnum<k34>, 10:w1673:i32[], 15:w1674:errorcluster)  [unwired: 3 in, 3 out]
              }
            }
            n154 = Index Array(array=w1639, index=0) -> (element=w1625:i32)
          }
          frame 18 {
            n155 = Build Array(w1692) -> (w1693:dbl[])
            n156 = TDMS List Contents(4:w1703, 6:w1705, 7:w1702) -> (0:w1709:errorcluster, 1:w1708:string[], 3:w1710:refnum<k34>)  [unwired: 1 out]
            n157 = Search 1D Array(1D array=w1708, element=w1704) -> (index of element=w1707:i32)  [unwired: 1 in]
            n158 = Greater Or Equal To 0?(x=w1707) -> (x >= 0?=w1706:bool)
            n159 = case shown="True" w1706 {
              tunnel: [w1724 w1729] -> w1700
              tunnel: [w1725 w1733] -> w1701
              tunnel: w1705 -> [_ w1727]
              tunnel: w1710 -> [w1725 w1732]
              tunnel: w1709 -> [w1724 w1731]
              tunnel: w1704 -> [_ w1726]
              tunnel: w1693 -> [w1723 w1730]
              tunnel: [w1723 w1728] -> w1695
              frame False {
              }
              frame True {
                n160 = TDMS Read(0:w1732, 5:w1727, 7:w1726, 11:w1731, 12:w1730) -> (4:w1733:refnum<k34>, 10:w1728:dbl[], 15:w1729:errorcluster)  [unwired: 3 in, 3 out]
              }
            }
            n161 = Index Array(array=w1695, index=0) -> (element=w1691:dbl)
          }
          frame 19 {
            n162 = TDMS List Contents(4:w1760, 6:w1762, 7:w1759) -> (0:w1766:errorcluster, 1:w1765:string[], 3:w1767:refnum<k34>)  [unwired: 1 out]
            n163 = Search 1D Array(1D array=w1765, element=w1761) -> (index of element=w1764:i32)  [unwired: 1 in]
            n164 = Greater Or Equal To 0?(x=w1764) -> (x >= 0?=w1763:bool)
            n165 = case shown="True" w1763 {
              tunnel: [w1776 w1781] -> w1757
              tunnel: [w1777 w1785] -> w1758
              tunnel: w1762 -> [_ w1779]
              tunnel: w1767 -> [w1777 w1784]
              tunnel: w1766 -> [w1776 w1783]
              tunnel: w1761 -> [_ w1780]
              tunnel: w1746 -> [w1775 w1782]
              tunnel: [w1775 w1778] -> w1745
              frame False {
              }
              frame True {
                n166 = TDMS Read(0:w1784, 5:w1779, 7:w1780, 11:w1783, 12:w1782) -> (4:w1785:refnum<k34>, 10:w1778:u16[], 15:w1781:errorcluster)  [unwired: 3 in, 3 out]
              }
            }
          }
          frame 20 {
            n167 = TDMS List Contents(4:w1812, 6:w1814, 7:w1811) -> (0:w1818:errorcluster, 1:w1817:string[], 3:w1819:refnum<k34>)  [unwired: 1 out]
            n168 = Search 1D Array(1D array=w1817, element=w1813) -> (index of element=w1816:i32)  [unwired: 1 in]
            n169 = Greater Or Equal To 0?(x=w1816) -> (x >= 0?=w1815:bool)
            n170 = case shown="True" w1815 {
              tunnel: [w1828 w1833] -> w1809
              tunnel: [w1829 w1837] -> w1810
              tunnel: w1814 -> [_ w1831]
              tunnel: w1819 -> [w1829 w1836]
              tunnel: w1818 -> [w1828 w1835]
              tunnel: w1813 -> [_ w1832]
              tunnel: w1798 -> [w1827 w1834]
              tunnel: [w1827 w1830] -> w1797
              frame False {
              }
              frame True {
                n171 = TDMS Read(0:w1836, 5:w1831, 7:w1832, 11:w1835, 12:w1834) -> (4:w1837:refnum<k34>, 10:w1830:dbl[], 15:w1833:errorcluster)  [unwired: 3 in, 3 out]
              }
            }
          }
          frame 21 {
            n172 = Build Array(w1849) -> (w1852:bool[])
            n173 = TDMS List Contents(4:w1862, 6:w1864, 7:w1861) -> (0:w1868:errorcluster, 1:w1867:string[], 3:w1869:refnum<k34>)  [unwired: 1 out]
            n174 = Search 1D Array(1D array=w1867, element=w1863) -> (index of element=w1866:i32)  [unwired: 1 in]
            n175 = Greater Or Equal To 0?(x=w1866) -> (x >= 0?=w1865:bool)
            n176 = case shown="True" w1865 {
              tunnel: [w1883 w1888] -> w1859
              tunnel: [w1884 w1892] -> w1860
              tunnel: w1864 -> [_ w1886]
              tunnel: w1869 -> [w1884 w1891]
              tunnel: w1868 -> [w1883 w1890]
              tunnel: w1863 -> [_ w1885]
              tunnel: w1852 -> [w1882 w1889]
              tunnel: [w1882 w1887] -> w1854
              frame False {
              }
              frame True {
                n177 = TDMS Read(0:w1891, 5:w1886, 7:w1885, 11:w1890, 12:w1889) -> (4:w1892:refnum<k34>, 10:w1887:bool[], 15:w1888:errorcluster)  [unwired: 3 in, 3 out]
              }
            }
            n178 = Index Array(array=w1854, index=0) -> (element=w1847:bool)
          }
          frame 22 {
            n179 = Build Array(w1903) -> (w1907:dbl[])
            n180 = TDMS List Contents(4:w1917, 6:w1919, 7:w1916) -> (0:w1923:errorcluster, 1:w1922:string[], 3:w1924:refnum<k34>)  [unwired: 1 out]
            n181 = Search 1D Array(1D array=w1922, element=w1918) -> (index of element=w1921:i32)  [unwired: 1 in]
            n182 = Greater Or Equal To 0?(x=w1921) -> (x >= 0?=w1920:bool)
            n183 = case shown="True" w1920 {
              tunnel: [w1938 w1943] -> w1914
              tunnel: [w1939 w1947] -> w1915
              tunnel: w1919 -> [_ w1941]
              tunnel: w1924 -> [w1939 w1946]
              tunnel: w1923 -> [w1938 w1945]
              tunnel: w1918 -> [_ w1940]
              tunnel: w1907 -> [w1937 w1944]
              tunnel: [w1937 w1942] -> w1909
              frame False {
              }
              frame True {
                n184 = TDMS Read(0:w1946, 5:w1941, 7:w1940, 11:w1945, 12:w1944) -> (4:w1947:refnum<k34>, 10:w1942:dbl[], 15:w1943:errorcluster)  [unwired: 3 in, 3 out]
              }
            }
            n185 = Index Array(array=w1909, index=0) -> (element=w1902:dbl)
          }
          frame 23 {
            n186 = Build Array(w1957) -> (w1955:u32[])
            n187 = TDMS List Contents(4:w1972, 6:w1974, 7:w1971) -> (0:w1978:errorcluster, 1:w1977:string[], 3:w1979:refnum<k34>)  [unwired: 1 out]
            n188 = Search 1D Array(1D array=w1977, element=w1973) -> (index of element=w1976:i32)  [unwired: 1 in]
            n189 = Greater Or Equal To 0?(x=w1976) -> (x >= 0?=w1975:bool)
            n190 = case shown="True" w1975 {
              tunnel: [w1993 w1998] -> w1969
              tunnel: [w1994 w2002] -> w1970
              tunnel: w1974 -> [_ w1996]
              tunnel: w1979 -> [w1994 w2001]
              tunnel: w1978 -> [w1993 w2000]
              tunnel: w1973 -> [_ w1995]
              tunnel: w1955 -> [w1992 w1999]
              tunnel: [w1992 w1997] -> w1964
              frame False {
              }
              frame True {
                n191 = TDMS Read(0:w2001, 5:w1996, 7:w1995, 11:w2000, 12:w1999) -> (4:w2002:refnum<k34>, 10:w1997:u32[], 15:w1998:errorcluster)  [unwired: 3 in, 3 out]
              }
            }
            n192 = Index Array(array=w1964, index=0) -> (element=w1956:u32)
          }
          frame 24 {
            n193 = Build Array(w2013) -> (w2011:string[])
            n194 = TDMS List Contents(4:w2027, 6:w2029, 7:w2026) -> (0:w2033:errorcluster, 1:w2032:string[], 3:w2034:refnum<k34>)  [unwired: 1 out]
            n195 = Search 1D Array(1D array=w2032, element=w2028) -> (index of element=w2031:i32)  [unwired: 1 in]
            n196 = Greater Or Equal To 0?(x=w2031) -> (x >= 0?=w2030:bool)
            n197 = case shown="True" w2030 {
              tunnel: [w2048 w2053] -> w2024
              tunnel: [w2049 w2057] -> w2025
              tunnel: w2029 -> [_ w2051]
              tunnel: w2034 -> [w2049 w2056]
              tunnel: w2033 -> [w2048 w2055]
              tunnel: w2028 -> [_ w2050]
              tunnel: w2011 -> [w2047 w2054]
              tunnel: [w2047 w2052] -> w2019
              frame False {
              }
              frame True {
                n198 = TDMS Read(0:w2056, 5:w2051, 7:w2050, 11:w2055, 12:w2054) -> (4:w2057:refnum<k34>, 10:w2052:string[], 15:w2053:errorcluster)  [unwired: 3 in, 3 out]
              }
            }
            n199 = Index Array(array=w2019, index=0) -> (element=w2010:string)
          }
          frame 26 {
            n200 = TDMS List Contents(4:w2079, 6:w2081, 7:w2078) -> (0:w2085:errorcluster, 1:w2084:string[], 3:w2086:refnum<k34>)  [unwired: 1 out]
            n201 = Search 1D Array(1D array=w2084, element=w2080) -> (index of element=w2083:i32)  [unwired: 1 in]
            n202 = Greater Or Equal To 0?(x=w2083) -> (x >= 0?=w2082:bool)
            n203 = case shown="True" w2082 {
              tunnel: [w2100 w2105] -> w2076
              tunnel: [w2101 w2109] -> w2077
              tunnel: w2081 -> [_ w2103]
              tunnel: w2086 -> [w2101 w2108]
              tunnel: w2085 -> [w2100 w2107]
              tunnel: w2080 -> [_ w2102]
              tunnel: w2064 -> [w2099 w2106]
              tunnel: [w2099 w2104] -> w2060
              frame False {
              }
              frame True {
                n204 = TDMS Read(0:w2108, 5:w2103, 7:w2102, 11:w2107, 12:w2106) -> (4:w2109:refnum<k34>, 10:w2104:dbl[], 15:w2105:errorcluster)  [unwired: 3 in, 3 out]
              }
            }
          }
          frame 27 {
            n205 = TDMS List Contents(4:w2131, 6:w2133, 7:w2130) -> (0:w2137:errorcluster, 1:w2136:string[], 3:w2138:refnum<k34>)  [unwired: 1 out]
            n206 = Search 1D Array(1D array=w2136, element=w2132) -> (index of element=w2135:i32)  [unwired: 1 in]
            n207 = Greater Or Equal To 0?(x=w2135) -> (x >= 0?=w2134:bool)
            n208 = case shown="True" w2134 {
              tunnel: [w2152 w2157] -> w2128
              tunnel: [w2153 w2161] -> w2129
              tunnel: w2133 -> [_ w2155]
              tunnel: w2138 -> [w2153 w2160]
              tunnel: w2137 -> [w2152 w2159]
              tunnel: w2132 -> [_ w2154]
              tunnel: w2114 -> [w2151 w2158]
              tunnel: [w2151 w2156] -> w2113
              frame False {
              }
              frame True {
                n209 = TDMS Read(0:w2160, 5:w2155, 7:w2154, 11:w2159, 12:w2158) -> (4:w2161:refnum<k34>, 10:w2156:dbl[], 15:w2157:errorcluster)  [unwired: 3 in, 3 out]
              }
            }
          }
          frame 28 {
            n210 = TDMS List Contents(4:w2183, 6:w2185, 7:w2182) -> (0:w2189:errorcluster, 1:w2188:string[], 3:w2190:refnum<k34>)  [unwired: 1 out]
            n211 = Search 1D Array(1D array=w2188, element=w2184) -> (index of element=w2187:i32)  [unwired: 1 in]
            n212 = Greater Or Equal To 0?(x=w2187) -> (x >= 0?=w2186:bool)
            n213 = case shown="True" w2186 {
              tunnel: [w2204 w2209] -> w2180
              tunnel: [w2205 w2213] -> w2181
              tunnel: w2185 -> [_ w2207]
              tunnel: w2190 -> [w2205 w2212]
              tunnel: w2189 -> [w2204 w2211]
              tunnel: w2184 -> [_ w2206]
              tunnel: w2166 -> [w2203 w2210]
              tunnel: [w2203 w2208] -> w2164
              frame False {
              }
              frame True {
                n214 = TDMS Read(0:w2212, 5:w2207, 7:w2206, 11:w2211, 12:w2210) -> (4:w2213:refnum<k34>, 10:w2208:dbl[], 15:w2209:errorcluster)  [unwired: 3 in, 3 out]
              }
            }
          }
        }
      }
      n215 = for {
        N: 4 -> [_]
        tunnel: w491 -> [w562]
        shift-right: [w554] -> w512
        shift-left: w513 -> [w555]
        shift-right: [w557] -> w492
        shift-left: w509 -> [w559]
        shift-right: [w560] -> w510
        shift-left: w508 -> [w558]
        shift-right: [w561] -> w511
        shift-left: _ -> [w553]
        shift-right: [w552] -> w490
        shift-left: _ -> [w551]
        i -> [w556]
        n216 = case shown="0, Default" w556 {
          tunnel: w562 -> [w563 w590]
          tunnel: [w578 w605] -> w561
          tunnel: [w565 w604] -> w560
          tunnel: w559 -> [w567 w603]
          tunnel: w558 -> [w568 w602]
          tunnel: [w566 w601] -> w557
          tunnel: w555 -> [w577 w592]
          tunnel: [w577 w592] -> w554
          tunnel: w553 -> [w578 _]
          tunnel: [w564 w591] -> w552
          tunnel: w551 -> [_ w591]
          frame 1 {
            n217 = TDMS List Contents(4:w567, 6:w563, 7:w568) -> (0:w570:errorcluster, 1:w574:string[], 3:w571:refnum<k34>)  [unwired: 1 out]
            n218 = Search 1D Array(1D array=w574, element="Hyb injection : buffer") -> (index of element=w575:i32)  [unwired: 1 in]
            n219 = Greater Or Equal To 0?(x=w575) -> (x >= 0?=w572:bool)
            n220 = case shown="True" w572 {
              tunnel: string[] ["Phot injection : pressure", "Phot injection : volume", "Phot injection : flow rate", "Phot injection : buffer"] ("channel name(s) in (Untitled)") -> [_ w588]
              tunnel: w571 -> [w579 w589]
              tunnel: w563 -> [_ w587]
              tunnel: w570 -> [w581 w586]
              tunnel: [w581 w585] -> w566
              tunnel: i32[][] [] ("Injection procedure IN hybridization") -> [w580 w584]
              tunnel: [w580 w583] -> w564
              tunnel: [w579 w582] -> w565
              frame False {
              }
              frame True {
                n221 = TDMS Read(0:w589, 5:w587, 7:w588, 11:w586, 12:w584) -> (4:w582:refnum<k34>, 10:w583:i32[][], 15:w585:errorcluster)  [unwired: 3 in, 3 out]
              }
            }
          }
          frame 0, Default {
            n222 = TDMS List Contents(4:w603, 6:w590, 7:w602) -> (0:w599:errorcluster, 1:w594:string[], 3:w598:refnum<k34>)  [unwired: 1 out]
            n223 = Search 1D Array(1D array=w594, element="Hyb injection : buffer") -> (index of element=w593:i32)  [unwired: 1 in]
            n224 = Greater Or Equal To 0?(x=w593) -> (x >= 0?=w596:bool)
            n225 = case shown="True" w596 {
              tunnel: string[] ["Hyb injection : pressure", "Hyb injection : volume", "Hyb injection : flow rate", "Hyb injection : buffer"] ("channel name(s) in (Untitled)") -> [_ w615]
              tunnel: w598 -> [w607 w616]
              tunnel: w590 -> [_ w614]
              tunnel: w599 -> [w608 w613]
              tunnel: [w608 w612] -> w601
              tunnel: [w607 w611] -> w604
              tunnel: i32[][] [] ("Injection procedure IN hybridization") -> [w606 w610]
              tunnel: [w606 w609] -> w605
              frame False {
              }
              frame True {
                n226 = TDMS Read(0:w616, 5:w614, 7:w615, 11:w613, 12:w610) -> (4:w611:refnum<k34>, 10:w609:i32[][], 15:w612:errorcluster)  [unwired: 3 in, 3 out]
              }
            }
          }
        }
      }
      n227 = String To Path(string=w483) -> (path=w482:path)
      n228 = Build Array(w532, w531, w479) -> (w530:dbl[][])
      n229 = Build Array(w528, w527, w526) -> (w525:dbl[][])
      n230 = Build Array(w523) -> (w499:string[][])
      n231 = Build Array(w521) -> (w496:string[][])
      n232 = Insert Into Array(array=w499, index (row)=w493, new element=w498) -> (w497:string[][])  [unwired: 1 in]
      n233 = Insert Into Array(array=w496, index (row)=w493, new element=w494) -> (w495:string[][])  [unwired: 1 in]
      n234 = Build Array(w476, w475, w474) -> (w477:dbl[][])
      n235 = Transpose 2D Array(2D array=w511) -> (transposed array=w535:i32[][])
      n236 = Transpose 2D Array(2D array=w490) -> (transposed array=w534:i32[][])
      n237 = Transpose 2D Array(2D array=w530) -> (transposed array=w529:dbl[][])
      n238 = Transpose 2D Array(2D array=w525) -> (transposed array=w524:dbl[][])
      n239 = Transpose 2D Array(2D array=w497) -> (transposed array=w522:string[][])
      n240 = Transpose 2D Array(2D array=w495) -> (transposed array=w520:string[][])
      n241 = Transpose 2D Array(2D array=w477) -> (transposed array=w473:dbl[][])
    }
  }
  "error out" <- w86
  n242 = To Single Precision Float(number=w49) -> (single precision float=w17:sgl[])
  n243 = To Long Integer(number=w63) -> (32bit integer=w75:i32[][])
  n244 = global write "Global_MAIN.vi" "tdms file out"(w85) -> ()
  n245 = for {
    tunnel: w75 -> [w2228] mode=indexing
    tunnel: [w2229] -> w72 mode=indexing
    i -> [w2224]
    n246 = Index Array(array=w2228, index #1=1 ("index"), index #2=0 ("index"), index #3=2 ("index")) -> (element #1=w2223:i32, element #2=w2222:i32, element #3=w2221:i32)
    n247 = call "RAMP_write_laser_line_item_name.vi"("Laser line number"=w2224, "Laser application"=w2221, "Power or time"=w2222, "Laser line"=w2223) -> ("Item name"=w2229:string)  [unwired: 1 in]
  }
  n248 = Index Array(array=w17, index #1=0 ("index"), index #2=1 ("index"), index #3=2 ("index"), index #4=3 ("index")) -> (element #1=w45:sgl, element #2=w44:sgl, element #3=w43:sgl, element #4=w15:sgl)
  n249 = Index Array(array=w34, index #1=0 ("index"), index #2=1 ("index"), index #3=2 ("index")) -> (element #1=w38:dbl, element #2=w39:dbl, element #3=w40:dbl)
  n250 = Array Size(array=w61) -> (size(s)=w60:i32[])
  n251 = To Unsigned Long Integer(number=w15) -> (unsigned 32bit integer=w14:u32)
  n252 = Bundle By Name(cluster=T4 {"proportional gain (Kc)"=15.0, "integral time (Ti, min)"=0.08, "derivative time (Td, min)"=0.0} ("PID gains"), "proportional gain (Kc)"=w38, "integral time (Ti, min)"=w39, "derivative time (Td, min)"=w40) -> (w5:T4)
  n253 = Index Array(array=w60, index=0) -> (element=w54:i32)
  n254 = Bundle By Name(cluster=T3 {"X"=0.0, "Y"=0.0, "SUM"=0.0, "count"=0} ("QPD ref"), "X"=w45, "Y"=w44, "SUM"=w43, "count"=w14) -> (w42:T3)
  n255 = Not Equal To 0?(x=w54) -> (x != 0?=w52:bool)
  n256 = Array Size(array=w57) -> (size(s)=w58:i32[])
  n257 = Index Array(array=w58, index=0) -> (element=w55:i32)
  n258 = Not Equal To 0?(x=w55) -> (x != 0?=w53:bool)
  n259 = Or(x=w53, y=w52) -> (x .or. y?=w50:bool)
  n260 = call "merFISH_define_injections_procedure_list_names.vi"("Buffer list"=w71, "Injection procedure IN photobleaching"=w57, "Injection procedure IN hybridization"=w61) -> ("Photobleaching name"=w73:string[], "Hybridization name"=w74:string[])  [unwired: 1 in, 2 out]
  n261 = Bundle By Name(cluster=w51, "Injection procedure defined"=w50) -> (w20:T5)
  n262 = Bundle By Name(cluster=T2 {"Hybridization name"=[], "Photobleaching name"=[], "Laser names"=[], "Buffer list names"=[], "Probe list names"=[]}, "Hybridization name"=w74, "Photobleaching name"=w73, "Laser names"=w72, "Buffer list names"=w71, "Probe list names"=w70) -> (→"Menu names cluster":T2)
  n263 = Bundle By Name(cluster=T1 {"Hybridization procedure"=[], "Photobleaching procedure"=[], "Alert email adress"="", "Exp time (s)"=0.0, "Total  range (nm)"=0, "step length (nm)"=0, "ROIs"=[], "Laser lines array"=[], "merFISH cluster"={"Autofocus calibrated"=FALSE, "Autofocus setpoint defined"=FALSE, "Laser defined"=FALSE, "ROI defined"=FALSE, "Injection procedure defined"=FALSE}, "Sample name"="", "FOV size"=0.0, "Mosaic size"=[], "PID gains"={"proportional gain (Kc)"=15.0, "integral time (Ti, min)"=0.08, "derivative time (Td, min)"=0.0}, "Illumination source"=TRUE, "Brightfield intensity"=0.0, "merFISH path"=path "", "QPD ref"={"X"=0.0, "Y"=0.0, "SUM"=0.0, "count"=0}, "REFs"=[], "N movies"=1, "N frames"=100}, "merFISH cluster"=w20, "Hybridization procedure"=w61, "Photobleaching procedure"=w57, "Alert email adress"=w68, "Exp time (s)"=w67, "Total  range (nm)"=w66, "step length (nm)"=w65, "ROIs"=w64, "Laser lines array"=w63, "QPD ref"=w42, "Sample name"=w41, "N movies"=w1, "N frames"=w2, "FOV size"=w3, "Mosaic size"=w4, "PID gains"=w5, "Illumination source"=w6, "Brightfield intensity"=w7, "merFISH path"=w8, "REFs"=w9) -> (→"Data cluster":T1)
